vi "SP_Read_Sensor.vi"() -> ()   [LabVIEW 2013]
uses:
  <vilib>/event_ctls.llb/eventvkey.ctl
  Global_Not-Aus.vi
  <vilib>/Utility/file.llb/Write To Spreadsheet File (DBL).vi
  <vilib>/Utility/file.llb/Read From Spreadsheet File (string).vi
  Global_Start_Stop_Einzelschritt.vi
panel:
  in  "Stop Program":bool
  in  "Port for KOSY3":refnum<visa-resource-name>="COM2"
  in  "Port for Powersupply":refnum<visa-resource-name>="COM3"
  in  "Port for Write Head":refnum<visa-resource-name>="COM4"
  in  "Port for ED33":refnum<visa-resource-name>="COM7"
  in  "Port for ED32i":refnum<visa-resource-name>="COM8"
  in  "X,Y,Z Value Limits":T1={"mm Xmin "=0.0, "mm Xmax "=100.0, " mm Ymin "=0.0, "mm Ymax "=267.9, " mm Zmin"=0.0, "mm Zmax "=108.0, "Schritte oder mm Umin (0)"=0.0, "Schritte oder mm Umax (0)"=0.0, "Schritte oder mm Cmin (0)"=0.0, "Schritte oder mm Cmax (0)"=0.0, "Schritte oder mm Amin (0)"=0.0, "Schritte oder mm Amax (0)"=0.0, "Schritte oder mm Bmin (0)"=0.0, "Schritte oder mm Bmax (0)"=0.0}
  out "Error Out":errorcluster caption="error out"
  in  "Error In":errorcluster caption="error in"
  out "Movement":T2={"Axis"=36, "Direction(To/From)"=0, "Speed in mm/s\n (5)[0,025-20]"=5.0, "IV6"=FALSE} {"Direction(To/From)" items=["vom Endschalter weg", "zum Endschalter hin"]; "Speed in mm/s\n (5)[0,025-20]" min=0.025 max=20; "Axis" items=["X-Achse"=36, "Y-Achse"=37, "Z-Achse"=38, "U-Achse"=63]}
  out "Keyboard Press Display":cluster{"Speed(+/-)":i16, "Movement":T3}
  out "Steps":dbl
  out "Current Sequence":string[](array[string])
  in  "Clear Sequence":bool
  in  "Load Sequence":bool
  out "Sequence":string[][](array[string])
  in  "File  Select":path
  in  "Activate Sequence?":bool
  in  "Tab Control":enum32{"Page 2"}(tab)
  in  "Main Tab":enum32{"Page 1", "Page 2"}(tab)
  in  "Multiple Control":enum32{"Position", "Sensors", "Results"}(tab)
  out "P6":dbl[](array[numeric])
  out "P5":dbl[](array[numeric])
  out "P4":dbl[](array[numeric])
  out "P3":dbl[](array[numeric])
  out "P7":dbl[](array[numeric])
  out "P2":dbl[](array[numeric])
  out "P1":dbl[](array[numeric])
  out "P8":dbl[](array[numeric])
  out "P9":dbl[](array[numeric])
  out "P10":dbl[](array[numeric])
  in  "Go To":bool
  in  "Position":T4(ring)
  in  "Save":bool
  in  "Reset All":bool
  in  "Reset":bool
  in  "Import":bool
  in  "File Path":path=path "Y:/01_Projekte/EPN93031_Schreibplatz/8_Konstruktionsunterlagen/8.5_Software/COPY_KOSY Steuerung LabVIEW/1.New_Code_2014_2015/2Pole_strip_Position.txt"
  in  "Export":bool
  out "Speed":dbl(knob) scale=0.0..10.0
  in  "Z axis":enum16{"Up", "Down"}(ring)
  in  "Y axis":enum16{"Forward", "Backward"}(ring)
  in  "X axis":enum16{"Left", "Right"}(ring)
  in  "Move Steps":bool
  in  "Steps(mm)":dbl[](array[numeric]) min=0.0
  in  "Count":dbl
  in  "Move & Measure":bool
  in  "ED33 Active?":bool
  in  "ED32i Active?":bool
  in  "Clear Sensor Readings":bool
  out "ED33_output":string[][](array[string])
  out "ED32i_output":string[][](array[string])
  out "ED32i":cluster{"Array 4[0]":i32, "Array 4[1]":i32}(graph)
  out "ED33":i32[](graph)
  out "Operation Done":string="Initialise"
  out "Current Status":string="Initialise"
  out "Moving":bool
  out "Stopped":bool
  in  "Home Position":bool
  out "Current Cordinates":T5 {"Schritte B" format="%#.4g"; "Schritte A" format="%#.4g"; "Schritte C" format="%#.4g"; "Schritte U" format="%#.4g"; "Z axis" format="%#.4g"; "Y axis" format="%#.4g"; "X axis" format="%#.4g"}
  # "Com port info"
  # "Instructions\n                                              Manual Control\n1. Run the program.\n2. Select 'Initialise' to start the program from first \n     or 'Continue' to continue the ongoing process.\n3. Select 'Normal Operation'.\n\nPolestrip Positions\n1. If already positions are already saved, select the corresponding \n    file in 'File Path' and then click 'Import' to get the corresponding\n    positions displayed on the front panel. \n2. Set the 'Speed' using (+/-) for the movement.\n3. Select a position from the dropdown 'Position'and click 'Go To'.\n    Else, \n1. Set the 'Speed' using (+/-) for the movement.\n2. Set the length for movement in 'Steps(mm)'  in corresponding \n    axis and also the direction of travel in the selected axis. \n    Then press 'Move'.\n3. Once desired position is reached, select a position from the \n    dropdown 'Position' and click 'Save'.\n4. Once all positions are saved in front panel, select the file  to be \n     saved in 'File Path' and click 'Export' to save positions to a text file.\n5. Select a position from the dropdown 'Position' and \n    Click 'Reset' to clear individual position.\n6. Click 'Reset All' to clear all positions.\n \nSensor Readings\nContinuous measurement\n1.Activate the sensor to be read from 'Read Sensors' tab.\n2.Set the length for movement in 'Steps(mm)' in corresponding \n    axis and also the direction of travel in the selected axis. \n    Then press 'Move'.\nMove and Measure\n1. Activate the sensor to be read from 'Read Sensors' tab.\n2.Set 'Count' to the number of times to measure.\n2.Set the length for movement in 'Steps(mm)' in corresponding \n    axis and also the direction of travel in the selected axis. \n    Then press 'Move Measure'.\n\n1. Click 'Clear' in 'Read Sensors' tab to clear the sensor readings.\n\n                                          Automatic Execution\n1. Run the program.\n2. Select 'Initialise' to start the program from first \n     or 'Continue' to continue the ongoing process.\n3. Select 'Normal Operation'.\n4. Select the corresponding file in 'File Select' and then click 'Load' \n    to get the corresponding codes in 'Sequence' .\n5. Click 'Clear' to clear sequence.\n6. Click 'Activate Sequence?' to run the automatic execution. \n\n                                                       General\n1. Click 'Stop Program' to stop the running program.\n2. Click 'Home Position' to take the write head to (0,0,0)."
  # "Instructions\n\n1. Positions are already saved, select the file in 'File Path' \n    and then 'Import' to get the positions displayed . \n2. Set the 'Speed' using (+/-) for the movement.\n3. Select a 'Position'and click 'Go To'.\n4. Click 'Reset All' to reset all positions and \n     'Import' again."
  # "Polestrip Positions"
  # "Instructions\n\nContinuous measurement\n1.Activate the sensor to be read.\n2.Set the length for movement in 'Steps(mm)' in corresponding \n    axis and also the direction of travel in the selected axis. \n    Then press 'Move'.\nMove and Measure\n1. Activate the sensor to be read.\n2.Set the length for movement in 'Steps(mm)' in corresponding \n    axis and also the direction of travel in the selected axis. \n3. Set 'Count' to the number of times to measure.  \n    Then press 'Move Measure'."
  # "[Click 'Clear' in 'Read Sensors' tab to clear the sensor readings.]"
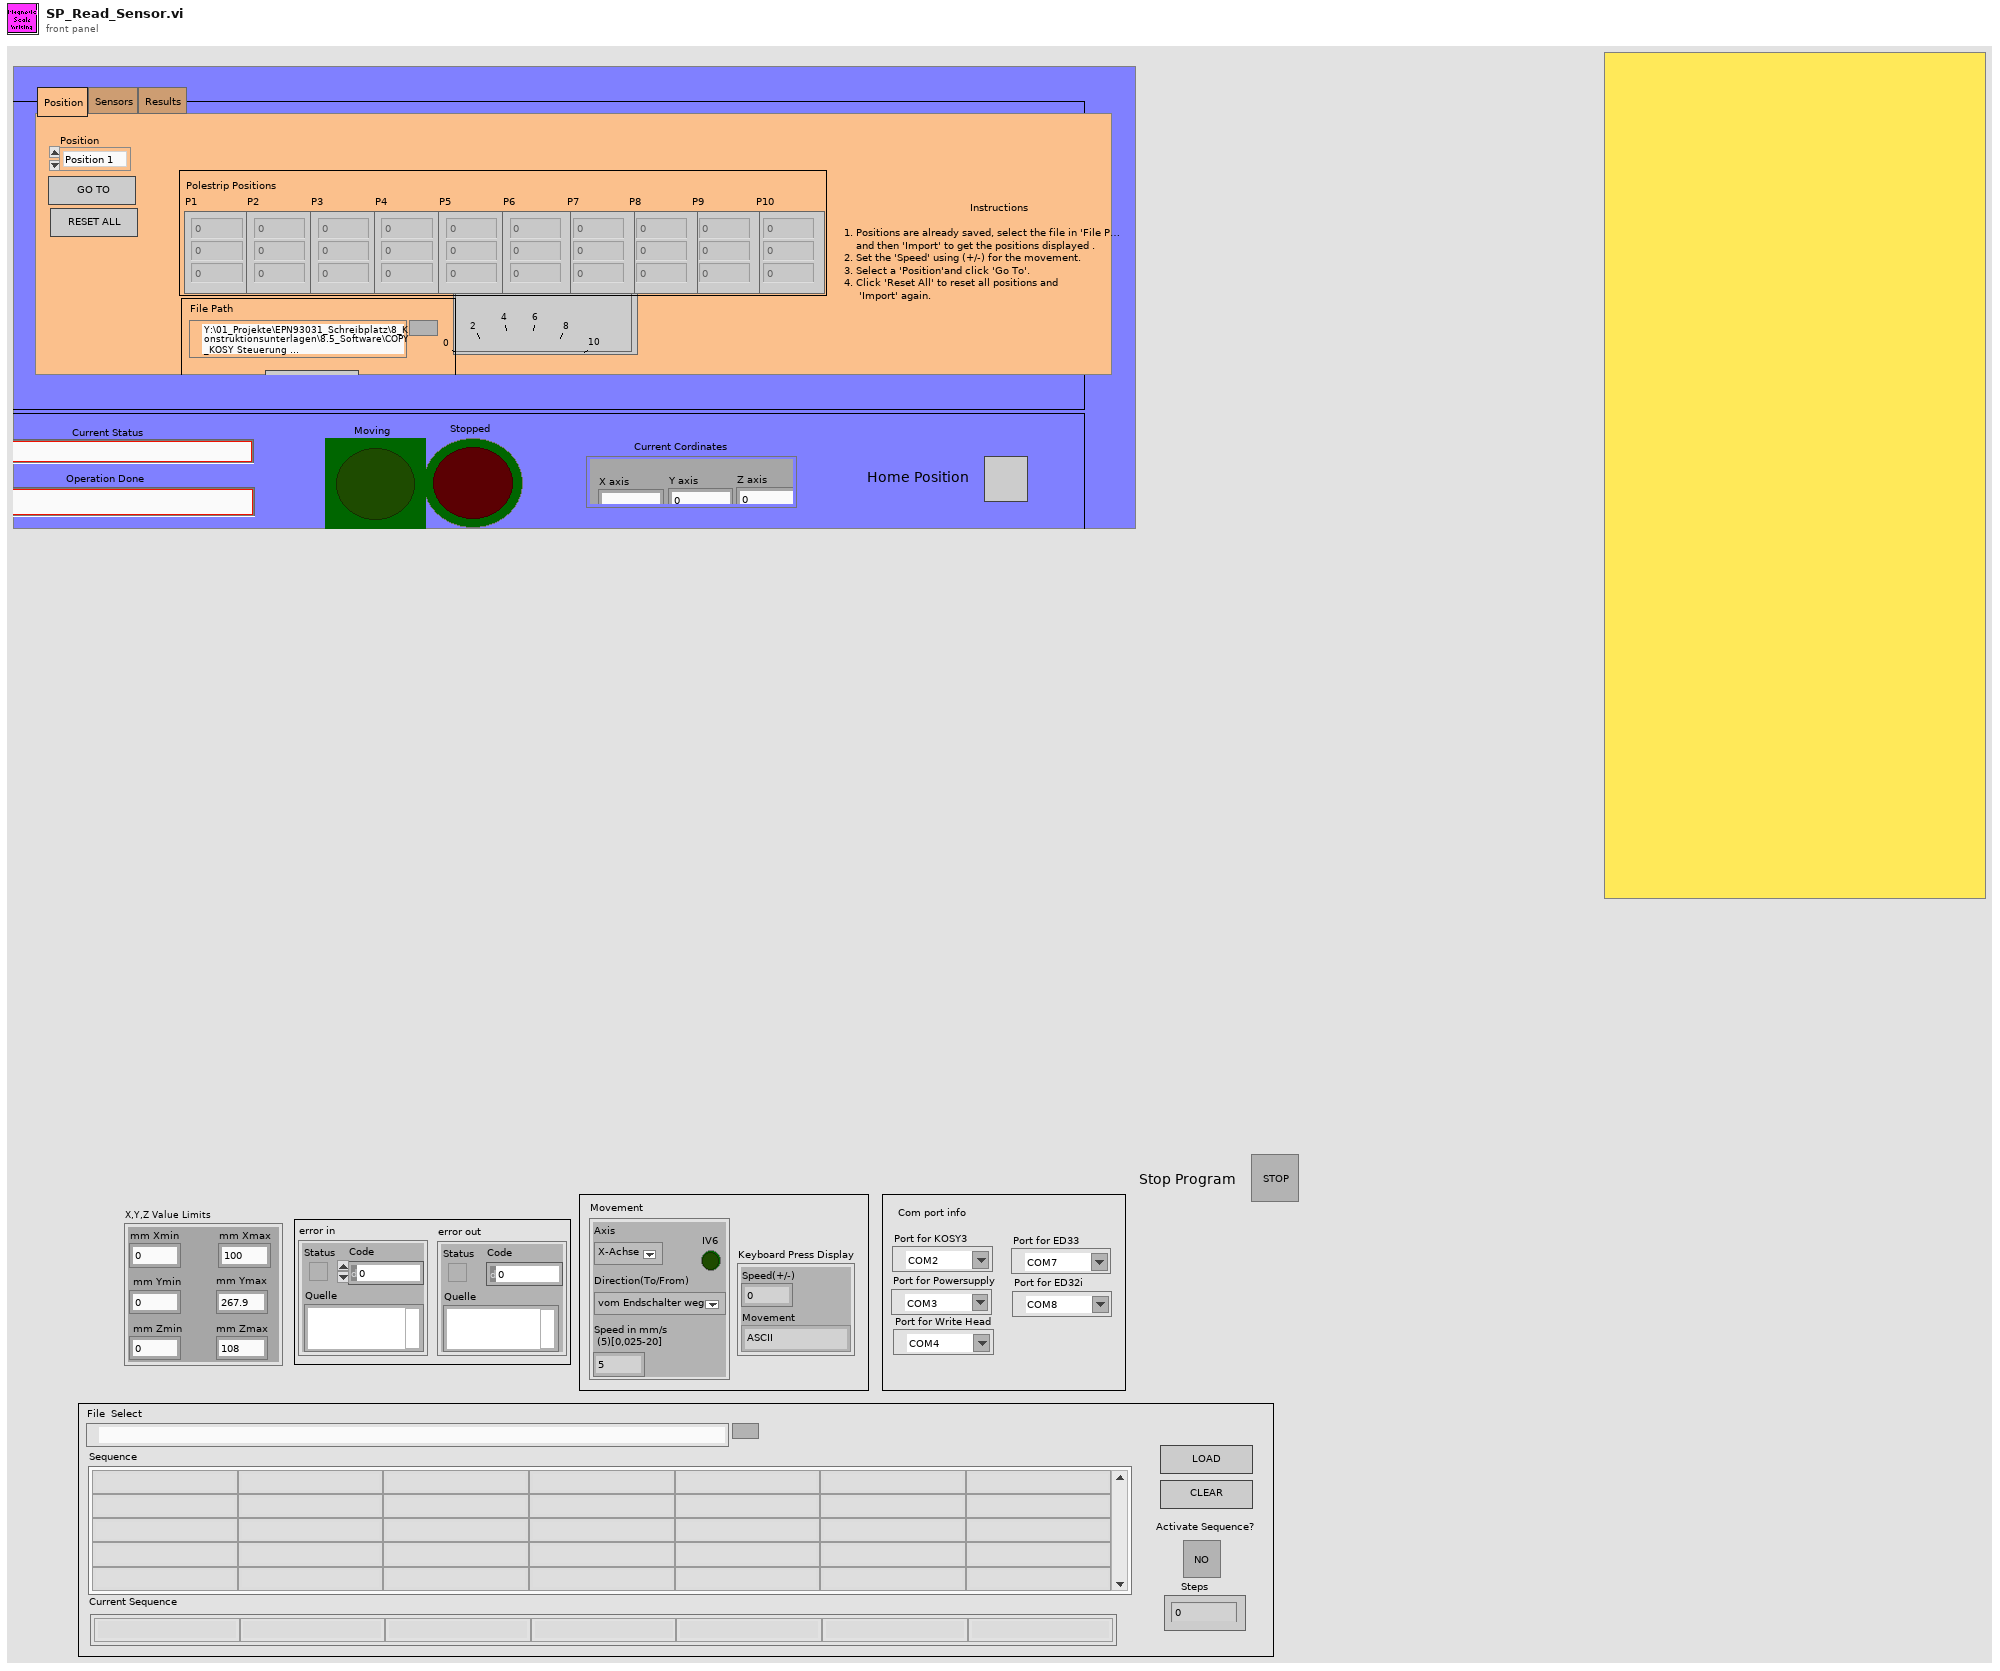
[diagram p1: front panel]
types:
  T1 = cluster{"mm Xmin ":sgl, "mm Xmax ":sgl, " mm Ymin ":sgl, "mm Ymax ":sgl, " mm Zmin":sgl, "mm Zmax ":sgl, "Schritte oder mm Umin (0)":sgl, "Schritte oder mm Umax (0)":sgl, "Schritte oder mm Cmin (0)":sgl, "Schritte oder mm Cmax (0)":sgl, "Schritte oder mm Amin (0)":sgl, "Schritte oder mm Amax (0)":sgl, "Schritte oder mm Bmin (0)":sgl, "Schritte oder mm Bmax (0)":sgl}
  T2 = cluster{"Axis":u8, "Direction(To/From)":u8, "Speed in mm/s\n (5)[0,025-20]":sgl, "IV6":bool}
  T3 = typedef "eventvkey.ctl" = enum16{"ASCII", "Enter", "Return", "Shift", "Ctrl", "Alt", "Cmd", "Opt", "Caps", "NumLock", "Clear", "Break", "Up", "Down", "Left", "Right", "Insert", "Delete", "Home", "End", "PageUp", "PageDown", "Escape", "Help", "Pause", "ScrollLock", "F1", "F2", "F3", "F4", "F5", "F6", "F7", "F8", "F9", "F10", "F11", "F12", "F13", "F14", "F15", "F16", "F17", "F18", "F19", "F20", "F21", "F22", "F23", "F24", "Play", "VolumeUp", "VolumeDown", "Mute", "Two Byte Char"}
  T4 = enum16{"Position 1", "Position 2", "Position 3", "Position 4", "Position 5", "Position 6", "Position 7", "Position 8", "Position 9", "Position 10"}
  T5 = cluster{"X axis":sgl, "Y axis":sgl, "Z axis":sgl, "Schritte U":sgl, "Schritte C":sgl, "Schritte A":sgl, "Schritte B":sgl}
  T6 = enum32{"Page Enabled", "Page Disabled", "Page Disabled & Grayed"}
  T7 = cluster{"Geschwindigkeit X in mm/s\n(5) [0,025-15]":sgl, "Geschwindigkeit Y in mm/s\n(5) [0,025-15]":sgl, "Geschwindigkeit Z in mm/s\n(5) [0,025-15]":sgl, "GeschwindigkeitU in mm/s\n(5) [0,025-15]":sgl}
  T8 = cluster{"Schritte X":sgl, "Schritte Y":sgl, "Schritte Z":sgl, "Schritte U":sgl, "Schritte C":sgl, "Schritte A":sgl, "Schritte B":sgl}
  T9 = cluster{"[0]":dbl, "[1]":dbl, "[2]":dbl, "[3]":dbl, "[4]":dbl, "[5]":dbl, "[6]":dbl, "[7]":dbl, "[8]":dbl}
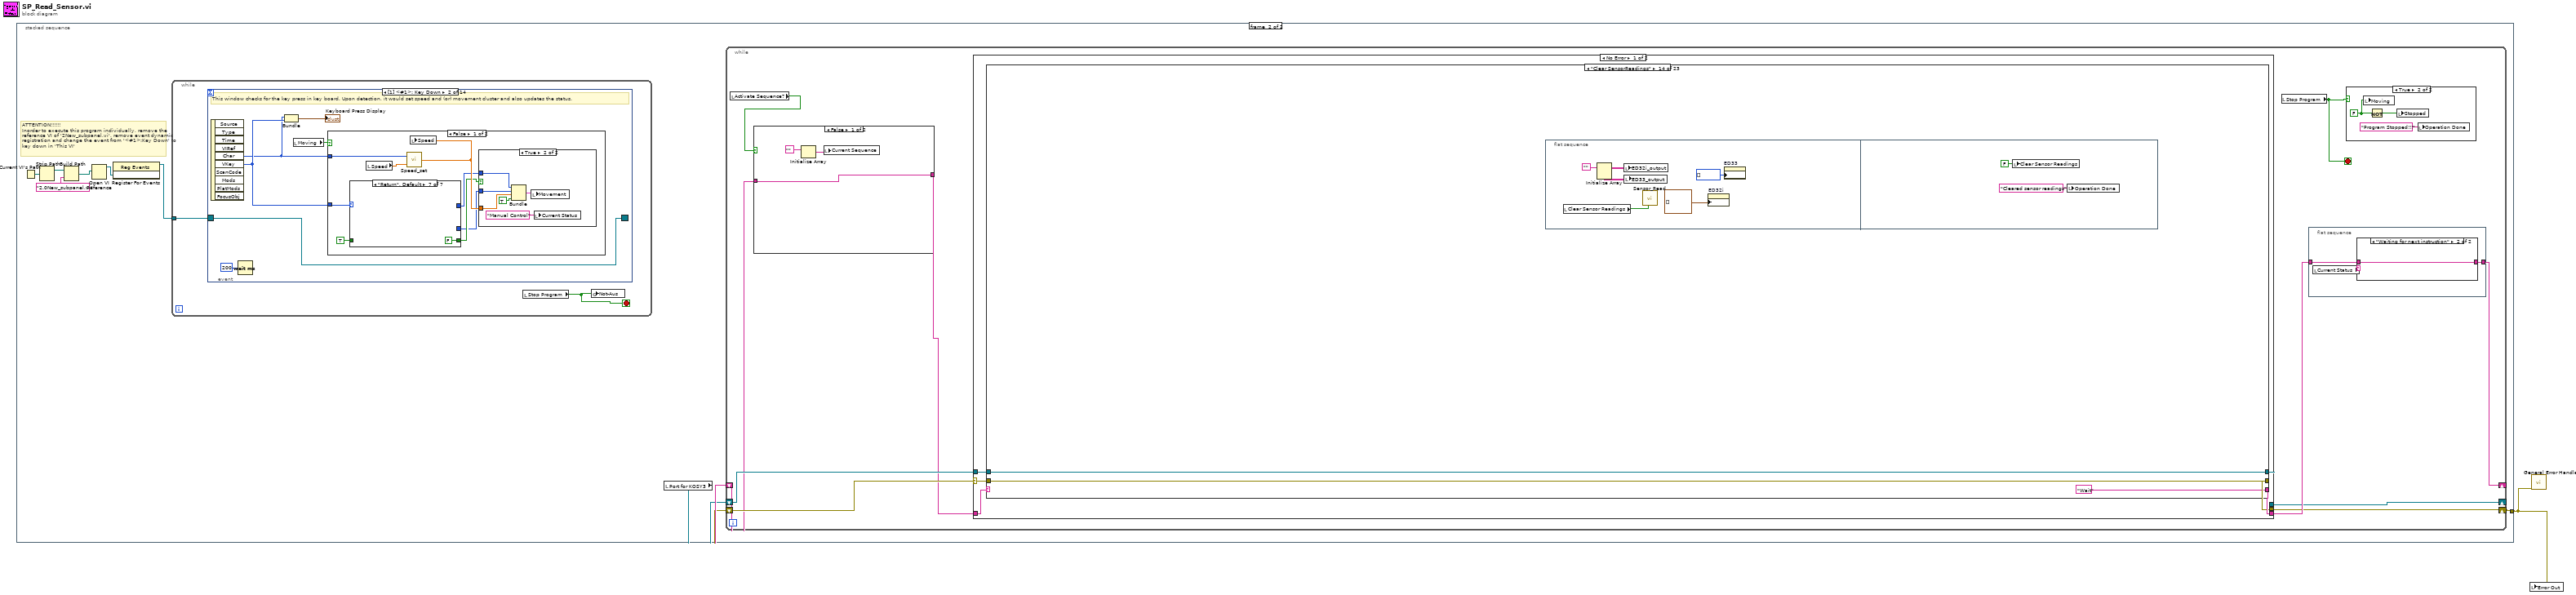
[diagram p0: block diagram]
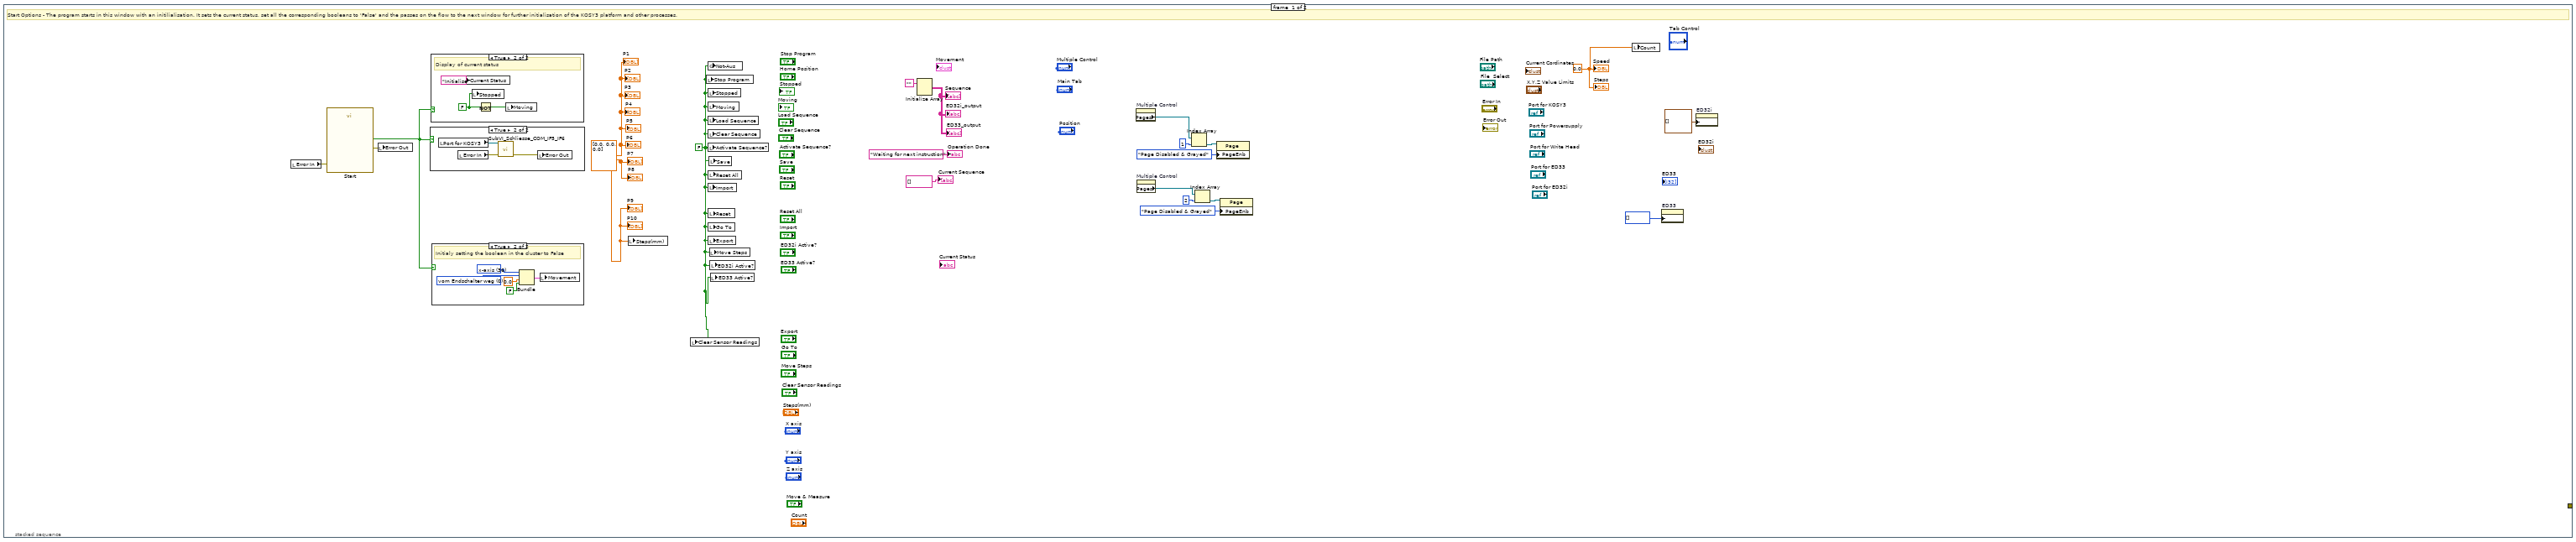
[diagram p2: hidden frame]
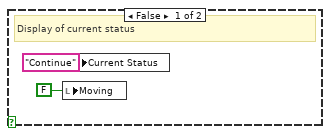
[diagram p5: hidden frame]
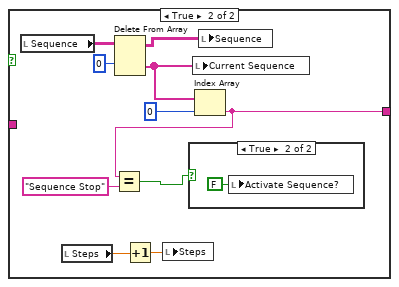
[diagram p6: hidden frame]
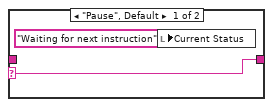
[diagram p9: hidden frame]
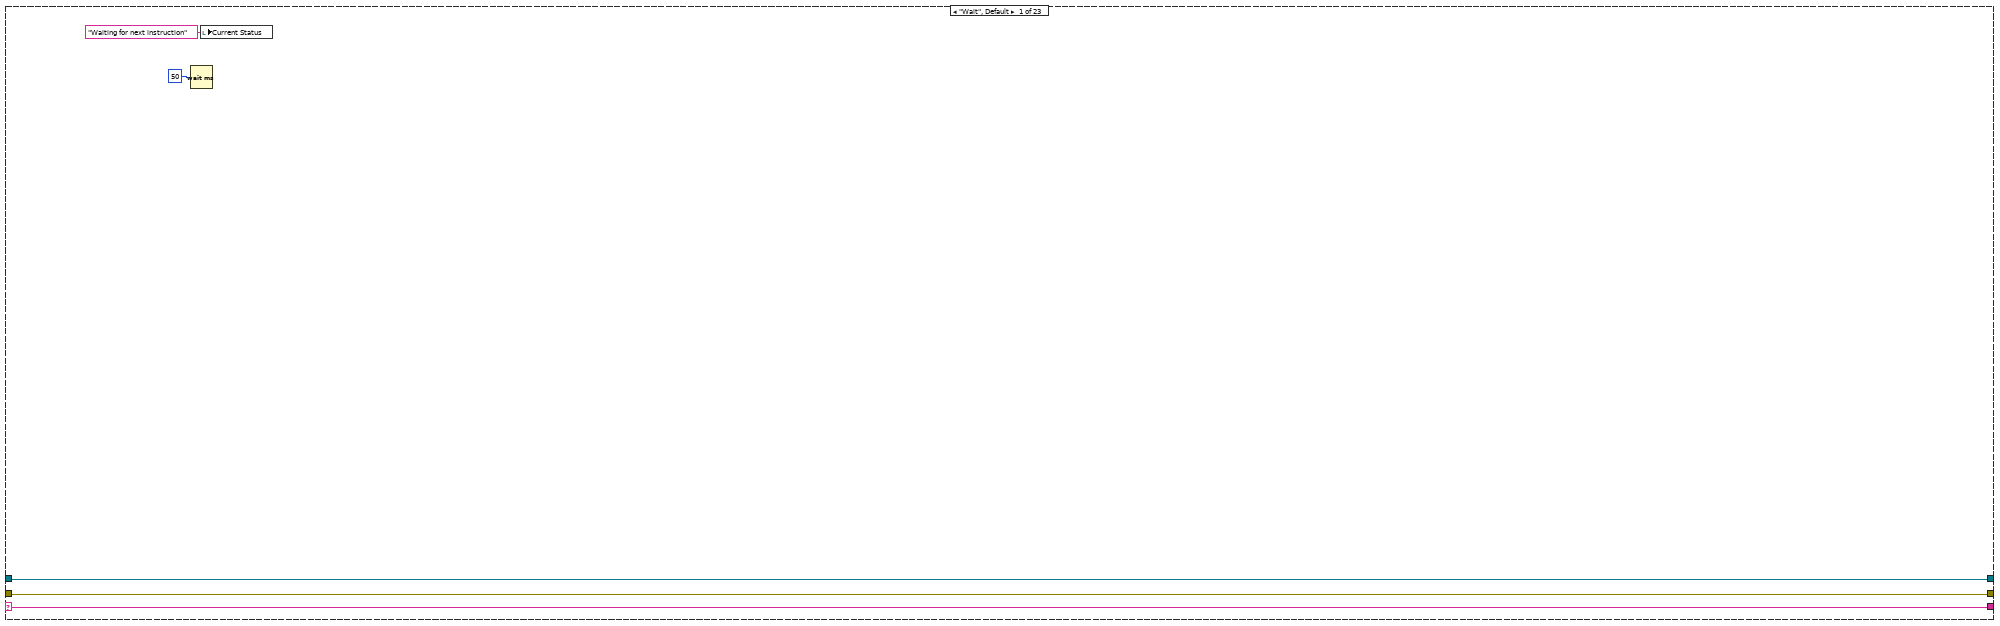
[diagram p10: hidden frame]
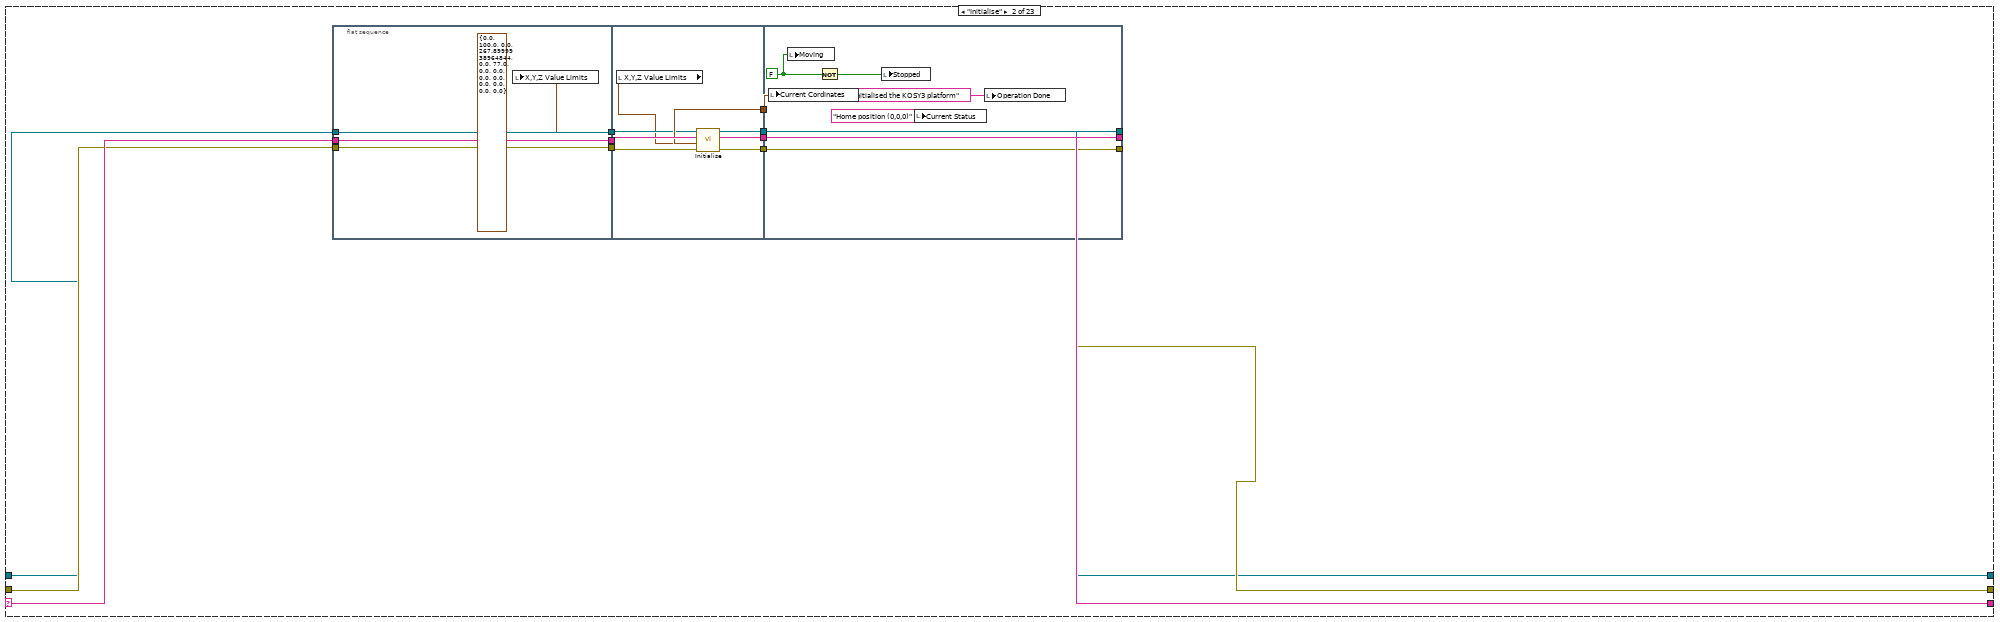
[diagram p11: hidden frame]
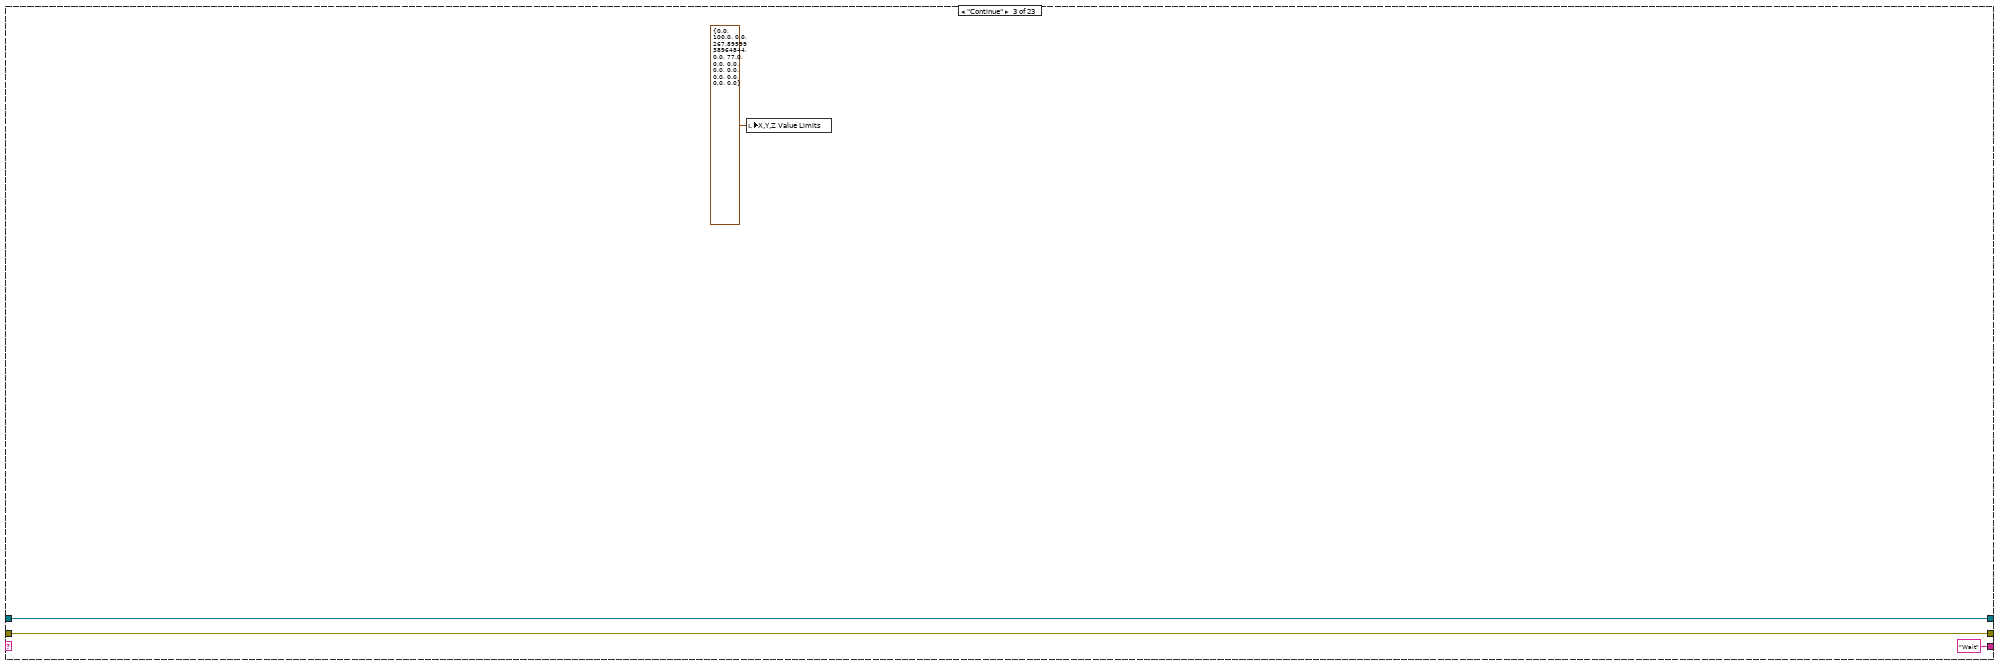
[diagram p12: hidden frame]
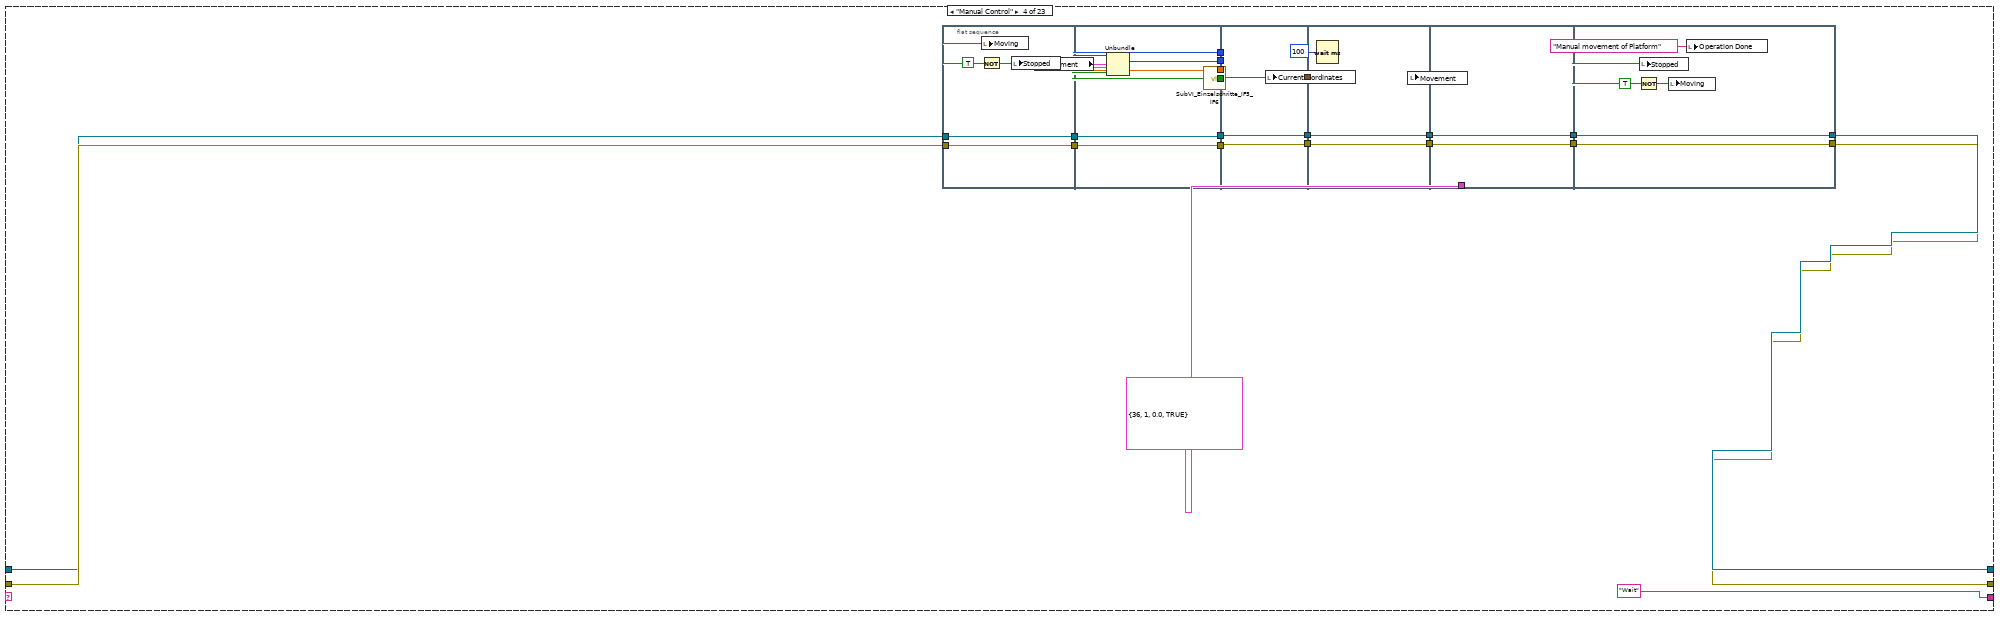
[diagram p13: hidden frame]
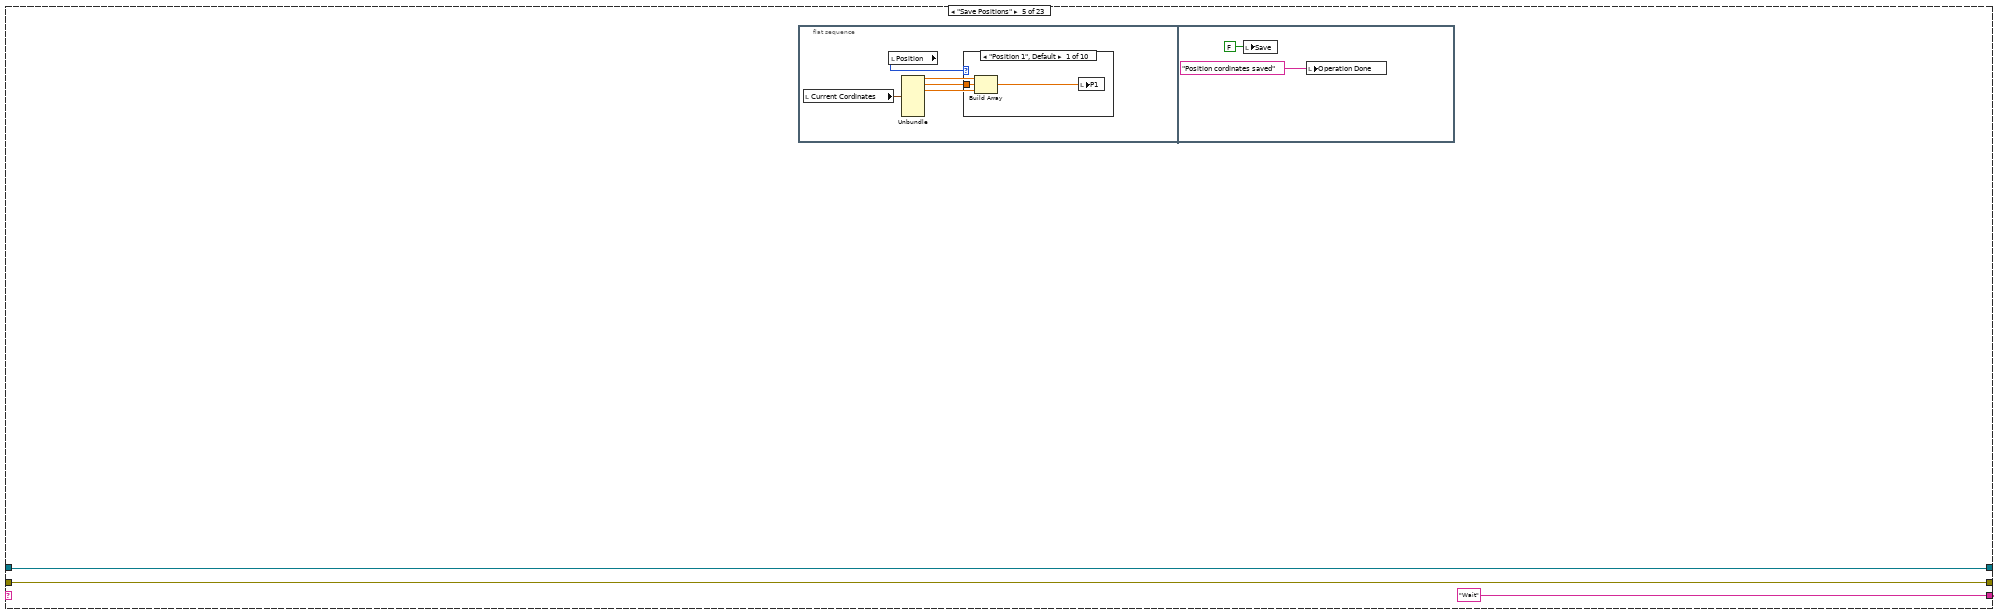
[diagram p14: hidden frame]
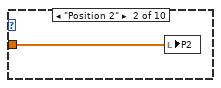
[diagram p15: hidden frame]
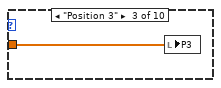
[diagram p16: hidden frame]
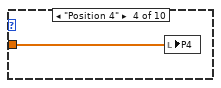
[diagram p17: hidden frame]
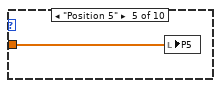
[diagram p18: hidden frame]
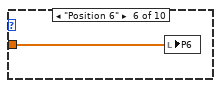
[diagram p19: hidden frame]
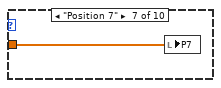
[diagram p20: hidden frame]
diagram:
  n1 = stacked-sequence {
    tunnel: [_ w41] -> w1
    frame #0 {
      w10 = 0.0 ("Speed")
      w11 = dbl[] [0.0, 0.0, 0.0] ("P1")
      w14 = FALSE ("Moving")
      # "Start Options - The program starts in this window with an initilialisation. It sets the current status, set all the corresponding booleans to 'False' and the passes on the flow to the next window for further initialisation of the KOSY3 platform and other processes."
      n2 = local read "Error In"() -> (w21:errorcluster)
      n3 = call "Start"("error in (no error)"=w21) -> ("Initialise"=w19:bool, "error out"=w20:errorcluster)  [unwired: 17 in]
      n4 = local write "Error Out"(w20) -> ()
      n5 = case shown="True" w19 {
        frame False {
        }
        frame True {
          n6 = local read "Port for KOSY3"() -> (w24:refnum<visa-resource-name>)
          n7 = local read "Error In"() -> (w23:errorcluster)
          n8 = call "SubVI_Schliesse_COM_IF5_IF6.vi"("VISA resource name in"=w24, "error in"=w23) -> ("error out"=w22:errorcluster)  [unwired: 13 in]
          n9 = local write "Error Out"(w22) -> ()
        }
      }
      n10 = case shown="True" w19 {
        frame False {
          # "Display of current status"
          n11 = local write "Moving"(FALSE ("Stopped")) -> ()
          n12 = local write "Current Status"("Continue") -> ()
        }
        frame True {
          w32 = FALSE ("Stopped")
          # "Display of current status"
          n13 = local write "Current Status"("Initialise") -> ()
          n14 = local write "Stopped"(w32) -> ()
          n15 = Not(x=w32) -> (.not. x?=w33:bool)
          n16 = local write "Moving"(w33) -> ()
        }
      }
      n17 = case shown="True" w19 {
        frame False {
        }
        frame True {
          w28 = u16 0 items=["vom Endschalter weg", "zum Endschalter hin"]
          w29 = u16 36 items=["x-axis"=36, "y-axis"=37, "z-axis"=38]
          # "Initialy setting the boolean in the cluster to False"
          n18 = Bundle(w29, w28, 0.0, FALSE) -> (w25:cluster{u16, u16, dbl, bool})  [unwired: 1 in]
          n19 = local write "Movement"(w25) -> ()
        }
      }
      n20 = local write "Steps(mm)"(w11) -> ()
      n21 = local write "Clear Sensor Readings"(w14) -> ()
      n22 = local write "Stop Program"(w14) -> ()
      n23 = global write "Global_Not-Aus.vi" "Not-Aus"(w14) -> ()
      n24 = local write "Stopped"(w14) -> ()
      n25 = local write "Moving"(w14) -> ()
      n26 = local write "Load Sequence"(w14) -> ()
      n27 = local write "Clear Sequence"(w14) -> ()
      n28 = local write "Activate Sequence?"(w14) -> ()
      n29 = local write "Import"(w14) -> ()
      n30 = local write "Reset All"(w14) -> ()
      n31 = local write "Reset"(w14) -> ()
      n32 = local write "Go To"(w14) -> ()
      n33 = local write "Export"(w14) -> ()
      n34 = local write "Save"(w14) -> ()
      n35 = local write "Move Steps"(w14) -> ()
      n36 = local write "ED32i Active?"(w14) -> ()
      n37 = local write "ED33 Active?"(w14) -> ()
      n38 = Initialize Array("" ("element")) -> (→"Sequence" →"ED32i_output" →"ED33_output":string[][])  [unwired: 2 in]
      n39 = property on="Multiple Control" class="TabCtl (strict)"() -> ("Pages"=w6:refnum<vi>[])  [unwired: 2 in, 2 out]
      n40 = property on="Multiple Control" class="TabCtl (strict)"() -> ("Pages"=w2:refnum<vi>[])  [unwired: 2 in, 2 out]
      n41 = Index Array(array=w6, index=1) -> (element=w7:refnum<vi>)
      n42 = Index Array(array=w2, index=2) -> (element=w3:refnum<vi>)
      n43 = property class="Page"(reference=w7, "PageEnb"=T6."Page Disabled & Grayed" ("Page Enabled State")) -> ()  [unwired: 1 in, 2 out]
      n44 = property class="Page"(reference=w3, "PageEnb"=T6."Page Disabled & Grayed" ("Page Enabled State")) -> ()  [unwired: 1 in, 2 out]
      n45 = local write "Count"(w10) -> ()
      n46 = property on="ED33" class="WFChart (strict)"("History Data"=i32[] []) -> ()  [unwired: 2 in, 2 out]
      n47 = property on="ED32i" class="WFChart (strict)"("History Data"=cluster{"Array 4[0]":i32, "Array 4[1]":i32}[] []) -> ()  [unwired: 2 in, 2 out]
      "Speed" <- w10
      "P1" <- w11
      "P2" <- w11
      "P3" <- w11
      "P7" <- w11
      "P4" <- w11
      "P5" <- w11
      "P6" <- w11
      "P8" <- w11
      "P9" <- w11
      "P10" <- w11
      "Current Sequence" <- string[] [] ("Current Sequence")
      "Operation Done" <- "Waiting for next instruction" ("Operation Done")
      "Steps" <- w10
    }
    frame #1 {
      # "ATTENTION!!!!!!\nInorder to execute this program individually, remove the reference VI of '2New_subpanel.vi', remove event dynamic registration and change the event from '<#1>:Key Down' to key down in 'This VI'"
      n48 = Current VI's Path() -> (path=w39:path)
      n49 = Strip Path(path=w39) -> (stripped path=w38:path)  [unwired: 1 out]
      n50 = Build Path(base path=w38, name or relative path="2.0New_subpanel.vi") -> (appended path=w36:path)
      n51 = Open VI Reference(vi path=w36) -> (vi reference=w40:refnum<vi>)  [unwired: 5 in, 1 out]
      n52 = register-events(w40) -> (reference out=w35:refnum<event-registration>)  [unwired: 2 in, 1 out]
      n53 = while {
        tunnel: w35 -> [w716]
        stop <- w717 stop-if-true
        n54 = event shown="[1] <#1>: Key Down" {
          selector: w716 -> [_ w719 _ _ _ _ _ _ _ _ _ _ _ _]
          dyn-events: [_ w719 _ _ _ _ _ _ _ _ _ _ _ _] -> _
          timeout: _ -> [_ _ _ _ _ _ _ _ _ _ _ _ _ _]
          event Timeout {
            n55 = event-data() -> ()  [unwired: 1 in, 2 out]
            n56 = global write "Global_Start_Stop_Einzelschritt.vi" "Boolesch"(FALSE ("Boolesch")) -> ()
          }
          event Key Down {
            # "This window checks for the key press in key board. Upon detection, it would set speed and (or) movement cluster and also updates the status."
            n57 = event-data() -> ("Char"=w720:i16, "VKey"=w722:T3)  [unwired: 1 in, 8 out]
            n58 = Wait (ms)(milliseconds to wait=u32 200) -> ()  [unwired: 1 out]
            n59 = Bundle("Char"=w720, "VKey"=w722) -> (→"Keyboard Press Display":cluster{"Char":i16, "VKey":T3})  [unwired: 1 in]
            n60 = local read "Moving"() -> (w724:bool)
            n61 = case shown="False" w724 {
              tunnel: w722 -> [w730 _]
              tunnel: w720 -> [w732 _]
              frame False {
                n62 = case shown="\"Return\", Default" w730 {
                  tunnel: [w733 w736 w739 w742 w745 w748 FALSE] -> w729
                  tunnel: [w735 w738 w741 w744 w747 w750 _] -> w727
                  tunnel: [w734 w737 w740 w743 w746 w749 _] -> w726
                  tunnel: TRUE -> [w733 w736 w739 w742 w745 w748 _]
                  frame "Left" {
                    w734 = u16 1 items=["vom Endschalter weg", "zum Endschalter hin"]
                    w735 = u16 36 items=["x-axis"=36, "y-axis"=37, "z-axis"=38]
                    # "Direction control(VKey identifies the directional keys)"
                  }
                  frame "Right" {
                    w737 = u16 0 items=["vom Endschalter weg", "zum Endschalter hin"]
                    w738 = u16 36 items=["x-axis"=36, "y-axis"=37, "z-axis"=38]
                    # "Direction control"
                  }
                  frame "Up" {
                    w740 = u16 1 items=["vom Endschalter weg", "zum Endschalter hin"]
                    w741 = u16 37 items=["x-axis"=36, "y-axis"=37, "z-axis"=38]
                    # "Direction control"
                  }
                  frame "Down" {
                    w743 = u16 0 items=["vom Endschalter weg", "zum Endschalter hin"]
                    w744 = u16 37 items=["x-axis"=36, "y-axis"=37, "z-axis"=38]
                  }
                  frame "PageUp" {
                    w746 = u16 1 items=["vom Endschalter weg", "zum Endschalter hin"]
                    w747 = u16 38 items=["x-axis"=36, "y-axis"=37, "z-axis"=38]
                  }
                  frame "PageDown" {
                    w749 = u16 0 items=["vom Endschalter weg", "zum Endschalter hin"]
                    w750 = u16 38 items=["x-axis"=36, "y-axis"=37, "z-axis"=38]
                  }
                  frame "Return", Default {
                  }
                }
                n63 = local read "Speed"() -> (w725:dbl)
                n64 = call "Speed_set.vi"("Speed"=w725, "Char"=w732) -> ("Speed"=w731:dbl)
                n65 = local write "Speed"(w731) -> ()
                n66 = case shown="True" w729 {
                  tunnel: w731 -> [_ w755]
                  tunnel: w727 -> [_ w754]
                  tunnel: w726 -> [_ w753]
                  frame False {
                  }
                  frame True {
                    n67 = Bundle(w754, w753, "Speed"=w755, TRUE) -> (w752:cluster{u16, u16, "Speed":dbl, bool})  [unwired: 1 in]
                    n68 = local write "Movement"(w752) -> ()
                    n69 = local write "Current Status"("Manual Control" ("Status")) -> ()
                  }
                }
              }
              frame True {
                n70 = global write "Global_Start_Stop_Einzelschritt.vi" "Boolesch"(TRUE) -> ()
                n71 = local write "Moving"(FALSE) -> ()
              }
            }
          }
          event "Home Position": Value Change {
            # "This window corresponds to the 'Home position' button on the Front Panel. Pressing the button will take KOSY3 paltform to the home position (0,0,0)"
            n72 = event-data() -> ()  [unwired: 1 in, 6 out]
            n73 = local write "Current Status"("Home Position" ("Status")) -> ()
          }
          event "Save": Value Change {
            # "When the 'SAVE' button in the Front Panel is pressed, it would save the current cordinates of the KOSY3 platform to the selected position."
            n74 = event-data() -> ()  [unwired: 1 in, 6 out]
            n75 = local write "Current Status"("Save Positions" ("Status")) -> ()
          }
          event "Reset": Value Change {
            # "When 'RESET' in the Front Panel is pressed, it resets the cordinates in the selected position to (0,0,0)"
            n76 = event-data() -> ()  [unwired: 1 in, 6 out]
            n77 = local write "Current Status"("Reset Position" ("Status")) -> ()
          }
          event "Reset All": Value Change {
            # "When 'RESET ALL' in the Front Panel is pressed, it resets the cordinates in all positions to (0,0,0)"
            n78 = event-data() -> ()  [unwired: 1 in, 6 out]
            n79 = local write "Current Status"("Reset All" ("Status")) -> ()
          }
          event "Go To": Value Change {
            n80 = event-data() -> ()  [unwired: 1 in, 6 out]
            n81 = local write "Current Status"("Go Position" ("Status")) -> ()
          }
          event "Move Steps": Value Change {
            n82 = event-data() -> ()  [unwired: 1 in, 6 out]
            n83 = local write "Current Status"("Go Straight" ("Status")) -> ()
          }
          event "Move & Measure": Value Change {
            n84 = event-data() -> ()  [unwired: 1 in, 6 out]
            n85 = local write "Current Status"("Move & Measure" ("Status")) -> ()
          }
          event "Import": Value Change {
            n86 = event-data() -> ()  [unwired: 1 in, 6 out]
            n87 = local write "Current Status"("Import Cordinates" ("Status")) -> ()
          }
          event "Export": Value Change {
            n88 = event-data() -> ()  [unwired: 1 in, 6 out]
            n89 = local write "Current Status"("Export Cordinates" ("Status")) -> ()
          }
          event "Load Sequence": Value Change {
            n90 = event-data() -> ()  [unwired: 1 in, 6 out]
            n91 = local write "Current Status"("Load Sequence" ("Status")) -> ()
          }
          event "Clear Sequence": Value Change {
            n92 = event-data() -> ()  [unwired: 1 in, 6 out]
            n93 = local write "Current Status"("Clear Sequence" ("Status")) -> ()
          }
          event "Clear Sensor Readings": Value Change {
            n94 = event-data() -> ()  [unwired: 1 in, 6 out]
            n95 = local write "Current Status"("Clear SensorReadings" ("Status")) -> ()
          }
        }
        n96 = local read "Stop Program"() -> (w717:bool)
        n97 = global write "Global_Not-Aus.vi" "Not-Aus"(w717) -> ()
      }
      n98 = local read "Port for KOSY3"() -> (w42:refnum<visa-resource-name>)
      n99 = local read "Current Status"() -> (w44:string)
      n100 = local read "Error In"() -> (w43:errorcluster)
      n101 = while {
        shift-right: [w48] -> w41
        shift-left: w43 -> [w54]
        shift-right: [w49] -> _
        shift-left: w42 -> [w50]
        shift-right: [w52] -> _
        shift-left: w44 -> [w47]
        stop <- w51 stop-if-true
        n102 = local read "Activate Sequence?"() -> (w45:bool)
        n103 = case shown="False" w45 {
          tunnel: w47 -> [w57 _]
          tunnel: [w57 w62] -> w46
          frame False {
            n104 = Initialize Array("") -> (w55:string[])  [unwired: 1 in]
            n105 = local write "Current Sequence"(w55) -> ()
          }
          frame True {
            n106 = local read "Sequence"() -> (w67:string[][])
            n107 = local read "Steps"() -> (w59:dbl)
            n108 = Delete From Array(array=w67, index (row)=0) -> (deleted portion=w64:string[], array with subset deleted=w65:string[][])  [unwired: 2 in]
            n109 = Increment(x=w59) -> (x+1=w58:dbl)
            n110 = local write "Steps"(w58) -> ()
            n111 = local write "Current Sequence"(w64) -> ()
            n112 = Index Array(array=w64, index=0) -> (element=w62:string)
            n113 = Equal?(x=w62, y="Sequence Stop") -> (x = y?=w60:bool)
            n114 = case shown="True" w60 {
              frame False {
              }
              frame True {
                n115 = local write "Activate Sequence?"(FALSE ("Activate Sequence?")) -> ()
              }
            }
            n116 = local write "Sequence"(w65) -> ()
          }
        }
        n117 = case shown="No Error" w54 {
          selector: w54 -> [w80 w711]
          tunnel: w46 -> [w83 _]
          tunnel: [w82 "Error" ("String 2")] -> w53
          tunnel: w50 -> [w81 w712]
          tunnel: [w78 w712] -> w49
          tunnel: [w79 w711] -> w48
          frame No Error {
            n118 = case shown="\"Clear SensorReadings\"" w83 {
              selector: w83 -> [w87 w101 _ _ _ _ _ _ _ _ _ _ _ _ _ _ _ _ _ _ _ _ _]
              tunnel: [w87 w98 "Wait" ("String 2") "Wait" "Wait" ("String 2") "Wait" ("String 2") "Wait" ("String 2") "Wait" ("String 2") "Wait" ("String 2") "Wait" ("String 2") "Wait" ("String 2") "Wait" ("String 2") "Wait" ("String 2") "Wait" ("String 2") "Wait" ("String 2") "Wait" ("String 2") "Wait" ("String 2") "Wait" ("String 2") "Wait" ("String 2") "Wait" ("String 2") "Wait" ("String 2") "Wait" ("String 2") "Wait" ("String 2")] -> w82
              tunnel: w81 -> [w84 w96 w124 w134 w180 w201 w218 w230 w268 w284 w323 w346 w353 w362 w371 w380 w394 w429 w556 w585 w593 w696 w703]
              tunnel: w80 -> [w85 w97 w122 w137 w179 w200 w217 w229 w269 w285 w325 w347 w354 w361 w372 w379 w395 w430 w554 w584 w594 w695 w705]
              tunnel: [w85 w94 w122 w129 w179 w200 w217 w227 w269 w285 w320 w347 w354 w361 w372 w379 w396 w428 w554 w584 w594 w695 w704] -> w79
              tunnel: [w84 w92 w124 w133 w180 w201 w218 w228 w268 w284 w322 w346 w353 w362 w371 w380 w397 w427 w556 w585 w592 w696 w703] -> w78
              frame "Wait", Default {
                n119 = Wait (ms)(milliseconds to wait=50) -> ()  [unwired: 1 out]
                n120 = local write "Current Status"("Waiting for next instruction" ("Status")) -> ()
              }
              frame "Initialise" {
                n121 = flat-sequence {
                  tunnel: w96 -> [w103]
                  tunnel: w97 -> [w104]
                  tunnel: w101 -> [w105]
                  tunnel: [w105] -> w91
                  tunnel: [w104] -> w90
                  tunnel: [w103] -> w89
                  tunnel: [w112] -> w100
                  tunnel: [w111] -> w99
                  tunnel: [w108] -> w95
                  tunnel: [w107] -> w93
                  tunnel: w91 -> [w113]
                  tunnel: w90 -> [w110]
                  tunnel: w89 -> [w109]
                  tunnel: w100 -> [w118]
                  tunnel: w99 -> [w117]
                  tunnel: [w117] -> w98
                  tunnel: [w115] -> w92
                  tunnel: w95 -> [w115]
                  tunnel: [w114] -> w94
                  tunnel: w93 -> [w114]
                  frame #0 {
                    n122 = local write "X,Y,Z Value Limits"(T1 {"mm Xmin "=0.0, "mm Xmax "=100.0, " mm Ymin "=0.0, "mm Ymax "=267.9, " mm Zmin"=0.0, "mm Zmax "=77.0, "Schritte oder mm Umin (0)"=0.0, "Schritte oder mm Umax (0)"=0.0, "Schritte oder mm Cmin (0)"=0.0, "Schritte oder mm Cmax (0)"=0.0, "Schritte oder mm Amin (0)"=0.0, "Schritte oder mm Amax (0)"=0.0, "Schritte oder mm Bmin (0)"=0.0, "Schritte oder mm Bmax (0)"=0.0} ("X,Y,Z Value Limits")) -> ()
                  }
                  frame #1 {
                    n123 = local read "X,Y,Z Value Limits"() -> (w106:T1)
                    n124 = call "Initialise.vi"("error IO"=w110, "X,Y,Z values"=w106, "String"=w113, "Port for KOSY3"=w109) -> ("Fehler (Ausgang)"=w107:errorcluster, "Cordinates of the  KOSY3 Platform"=w112:T8, "String 2"=w111:string, "VISA-Referenz (Ausgang)"=w108:refnum<visa-resource-name>)
                  }
                  frame #2 {
                    w119 = FALSE ("Stopped")
                    n125 = local write "Current Cordinates"(w118) -> ()
                    n126 = local write "Moving"(w119) -> ()
                    n127 = Not(x=w119) -> (.not. x?=w120:bool)
                    n128 = local write "Stopped"(w120) -> ()
                    n129 = local write "Current Status"("Home position (0,0,0)" ("Status")) -> ()
                    n130 = local write "Operation Done"("Initialised the KOSY3 platform" ("Operation Done")) -> ()
                  }
                }
              }
              frame "Continue" {
                n131 = local write "X,Y,Z Value Limits"(T1 {"mm Xmin "=0.0, "mm Xmax "=100.0, " mm Ymin "=0.0, "mm Ymax "=267.9, " mm Zmin"=0.0, "mm Zmax "=77.0, "Schritte oder mm Umin (0)"=0.0, "Schritte oder mm Umax (0)"=0.0, "Schritte oder mm Cmin (0)"=0.0, "Schritte oder mm Cmax (0)"=0.0, "Schritte oder mm Amin (0)"=0.0, "Schritte oder mm Amax (0)"=0.0, "Schritte oder mm Bmin (0)"=0.0, "Schritte oder mm Bmax (0)"=0.0} ("X,Y,Z Value Limits")) -> ()
              }
              frame "Manual Control" {
                n132 = flat-sequence {
                  tunnel: [w148] -> w138
                  tunnel: w137 -> [w148]
                  tunnel: [w147] -> w135
                  tunnel: w134 -> [w147]
                  tunnel: [w156] -> w145
                  tunnel: [w155] -> w144
                  tunnel: [w154] -> w143
                  tunnel: [w153] -> w142
                  tunnel: [w152] -> w139
                  tunnel: w138 -> [w152]
                  tunnel: [w151] -> w136
                  tunnel: w135 -> [w151]
                  tunnel: [w166] -> w141
                  tunnel: w145 -> [w165]
                  tunnel: w144 -> [w164]
                  tunnel: w143 -> [w163]
                  tunnel: w142 -> [w162]
                  tunnel: w139 -> [w161]
                  tunnel: w136 -> [w158]
                  tunnel: [w160] -> w130
                  tunnel: [w159] -> w126
                  tunnel: w141 -> [w169]
                  tunnel: [w168] -> w131
                  tunnel: w130 -> [w168]
                  tunnel: [w167] -> w127
                  tunnel: w126 -> [w167]
                  tunnel: cluster{u16, u16, dbl, bool} {36, 1, 0.0, TRUE} -> [w173]
                  tunnel: [w172] -> w132
                  tunnel: w131 -> [w172]
                  tunnel: [w171] -> w128
                  tunnel: w127 -> [w171]
                  tunnel: [w175] -> w133
                  tunnel: w132 -> [w175]
                  tunnel: [w174] -> w129
                  tunnel: w128 -> [w174]
                  frame #0 {
                    w149 = TRUE ("Moving")
                    n133 = Not(x=w149) -> (.not. x?=w150:bool)
                    n134 = local write "Moving"(w149) -> ()
                    n135 = local write "Stopped"(w150) -> ()
                  }
                  frame #1 {
                    n136 = local read "Movement"() -> (w157:T2)
                    n137 = Unbundle(w157) -> ("Axis"=w156:u8, "Direction(To/From)"=w155:u8, "Speed in mm/s\n (5)[0,025-20]"=w154:sgl, "IV6"=w153:bool)
                  }
                  frame #2 {
                    n138 = call <userlib>:"SubVI_Einzelschritte_IF5_IF6.vi"("VISA resource name in"=w158, "Achsen-Wahl (X)"=w165, "Geschwindigkeit\nin mm/s (5)[0,025-20]"=w163, "IF5=F/IF6=T\n(IF6=T) in"=w162, "error in"=w161, "Richtung (vEw)"=w164) -> ("VISA resource name out"=w160:refnum<visa-resource-name>, "Koordinaten IF6"=w166:T8, "error out"=w159:errorcluster)  [unwired: 3 in, 4 out]
                  }
                  frame #3 {
                    n139 = local write "Current Cordinates"(w169) -> ()
                    n140 = Wait (ms)(milliseconds to wait=u32 100) -> ()  [unwired: 1 out]
                  }
                  frame #4 {
                    n141 = local write "Movement"(w173) -> ()
                  }
                  frame #5 {
                    w178 = TRUE ("Moving")
                    n142 = Not(x=w178) -> (.not. x?=w177:bool)
                    n143 = local write "Stopped"(w178) -> ()
                    n144 = local write "Moving"(w177) -> ()
                    n145 = local write "Operation Done"("Manual movement of Platform" ("Status")) -> ()
                  }
                }
              }
              frame "Save Positions" {
                n146 = flat-sequence {
                  frame #0 {
                    n147 = local read "Current Cordinates"() -> (w185:T5)
                    n148 = local read "Position"() -> (w187:T4)
                    n149 = Unbundle(w185) -> ("X axis"=w182:sgl, "Y axis"=w183:sgl, "Z axis"=w184:sgl)  [unwired: 4 out]
                    n150 = Build Array(w182, w183, w184) -> (w186:sgl[])
                    n151 = case shown="\"Position 1\", Default" w187 {
                      tunnel: w186 -> [w188 w189 w190 w191 w192 w193 w194 w195 w196 w197]
                      frame "Position 1", Default {
                        n152 = local write "P1"(w188) -> ()
                      }
                      frame "Position 2" {
                        n153 = local write "P2"(w189) -> ()
                      }
                      frame "Position 3" {
                        n154 = local write "P3"(w190) -> ()
                      }
                      frame "Position 4" {
                        n155 = local write "P4"(w191) -> ()
                      }
                      frame "Position 5" {
                        n156 = local write "P5"(w192) -> ()
                      }
                      frame "Position 6" {
                        n157 = local write "P6"(w193) -> ()
                      }
                      frame "Position 7" {
                        n158 = local write "P7"(w194) -> ()
                      }
                      frame "Position 8" {
                        n159 = local write "P8"(w195) -> ()
                      }
                      frame "Position 9" {
                        n160 = local write "P9"(w196) -> ()
                      }
                      frame "Position 10" {
                        n161 = local write "P10"(w197) -> ()
                      }
                    }
                  }
                  frame #1 {
                    n162 = local write "Save"(FALSE ("Save Button")) -> ()
                    n163 = local write "Operation Done"("Position cordinates saved" ("Operation Done")) -> ()
                  }
                }
              }
              frame "Reset Position" {
                n164 = flat-sequence {
                  frame #0 {
                    n165 = local read "Position"() -> (w203:T4)
                    n166 = case shown="\"Position 10\"" w203 {
                      tunnel: dbl[] [0.0, 0.0, 0.0] ("P1") -> [w205 w206 w207 w208 w209 w210 w211 w212 w213 w214]
                      frame "Position 1", Default {
                        n167 = local write "P1"(w205) -> ()
                      }
                      frame "Position 2" {
                        n168 = local write "P2"(w206) -> ()
                      }
                      frame "Position 3" {
                        n169 = local write "P3"(w207) -> ()
                      }
                      frame "Position 4" {
                        n170 = local write "P4"(w208) -> ()
                      }
                      frame "Position 5" {
                        n171 = local write "P5"(w209) -> ()
                      }
                      frame "Position 6" {
                        n172 = local write "P6"(w210) -> ()
                      }
                      frame "Position 7" {
                        n173 = local write "P7"(w211) -> ()
                      }
                      frame "Position 8" {
                        n174 = local write "P8"(w212) -> ()
                      }
                      frame "Position 9" {
                        n175 = local write "P9"(w213) -> ()
                      }
                      frame "Position 10" {
                        n176 = local write "P10"(w214) -> ()
                      }
                    }
                  }
                  frame #1 {
                    n177 = local write "Reset"(FALSE ("Reset")) -> ()
                    n178 = local write "Operation Done"("The selected position is reset" ("Operation Done")) -> ()
                  }
                }
              }
              frame "Reset All" {
                n179 = flat-sequence {
                  frame #0 {
                    w220 = dbl[] [0.0, 0.0, 0.0] ("P1")
                    n180 = local write "P1"(w220) -> ()
                    n181 = local write "P2"(w220) -> ()
                    n182 = local write "P3"(w220) -> ()
                    n183 = local write "P4"(w220) -> ()
                    n184 = local write "P5"(w220) -> ()
                    n185 = local write "P6"(w220) -> ()
                    n186 = local write "P7"(w220) -> ()
                    n187 = local write "P8"(w220) -> ()
                    n188 = local write "P9"(w220) -> ()
                    n189 = local write "P10"(w220) -> ()
                    n190 = local write "Steps(mm)"(w220) -> ()
                  }
                  frame #1 {
                    n191 = local write "Reset All"(FALSE ("Reset all Positions")) -> ()
                    n192 = local write "Operation Done"("Reset all positions" ("Operation Done")) -> ()
                  }
                }
              }
              frame "Go Position" {
                n193 = flat-sequence {
                  tunnel: [w235] -> w226
                  tunnel: [w234] -> w225
                  tunnel: w230 -> [w237]
                  tunnel: w229 -> [w236]
                  tunnel: w226 -> [w261]
                  tunnel: w225 -> [w260]
                  tunnel: [w261] -> w224
                  tunnel: [w260] -> w223
                  tunnel: [w266] -> w227
                  tunnel: [w267] -> w228
                  tunnel: w224 -> [w267]
                  tunnel: w223 -> [w266]
                  frame #0 {
                    w233 = TRUE ("Moving")
                    n194 = local write "Moving"(w233) -> ()
                    n195 = local read "Position"() -> (w245:T4)
                    n196 = case shown="\"Position 10\"" w245 {
                      tunnel: [w246 w247 w248 w249 w250 w251 w252 w253 w254 w255] -> w243
                      frame "Position 1", Default {
                        n197 = local read "P1"() -> (w246:dbl[])
                      }
                      frame "Position 2" {
                        n198 = local read "P2"() -> (w247:dbl[])
                      }
                      frame "Position 3" {
                        n199 = local read "P3"() -> (w248:dbl[])
                      }
                      frame "Position 4" {
                        n200 = local read "P4"() -> (w249:dbl[])
                      }
                      frame "Position 5" {
                        n201 = local read "P5"() -> (w250:dbl[])
                      }
                      frame "Position 6" {
                        n202 = local read "P6"() -> (w251:dbl[])
                      }
                      frame "Position 7" {
                        n203 = local read "P7"() -> (w252:dbl[])
                      }
                      frame "Position 8" {
                        n204 = local read "P8"() -> (w253:dbl[])
                      }
                      frame "Position 9" {
                        n205 = local read "P9"() -> (w254:dbl[])
                      }
                      frame "Position 10" {
                        n206 = local read "P10"() -> (w255:dbl[])
                      }
                    }
                    n207 = Not(x=w233) -> (.not. x?=w232:bool)
                    n208 = local write "Stopped"(w232) -> ()
                    n209 = local read "Speed"() -> (w239:dbl)
                    n210 = local read "Current Cordinates"() -> (w242:T5)
                    n211 = Bundle(0, "Speed"=w239, 0) -> (w238:cluster{i32, "Speed":dbl, i32})  [unwired: 1 in]
                    n212 = call <userlib>:"SubVI_Punkt_anfahren_IF5_IF6.vi"("Angehängtes Array"=w243, "error in"=w236, "Koordinaten in IF6"=w242, "Geschwindigkeiten"=w238, "VISA resource name in"=w237) -> ("error out"=w234:errorcluster, "Koordinaten out IF6"=w244:T8, "VISA resource name in 2"=w235:refnum<visa-resource-name>)  [unwired: 1 in]
                    n213 = local write "Current Cordinates"(w244) -> ()
                  }
                  frame #1 {
                    w256 = TRUE ("Moving")
                    n214 = local write "Go To"(FALSE ("Go To")) -> ()
                    n215 = local write "Stopped"(w256) -> ()
                    n216 = Not(x=w256) -> (.not. x?=w257:bool)
                    n217 = local write "Moving"(w257) -> ()
                    n218 = local write "Operation Done"("Go to the selected position" ("Operation Done")) -> ()
                  }
                  frame #2 {
                    n219 = property on="Multiple Control" class="TabCtl (strict)"() -> ("Pages"=w262:refnum<vi>[])  [unwired: 2 in, 2 out]
                    n220 = Index Array(array=w262, index=1) -> (element=w263:refnum<vi>)
                    n221 = property class="Page"(reference=w263, "PageEnb"=T6."Page Enabled" ("Page Enabled State")) -> ()  [unwired: 1 in, 2 out]
                  }
                }
              }
              frame "Import Cordinates" {
                n222 = flat-sequence {
                  frame #0 {
                    n223 = local read "File Path"() -> (w281:path)
                    n224 = call "Dekoder Batch Speicher.vi"("Batchfeld Speicher"=w281) -> ("P9"=w271:dbl[], "P10"=w272:dbl[], "P1"=w273:dbl[], "P2"=w274:dbl[], "P8"=w275:dbl[], "P3"=w276:dbl[], "P4"=w277:dbl[], "P7"=w280:dbl[], "P6"=w278:dbl[], "P5"=w279:dbl[])  [unwired: 5 in]
                    n225 = local write "P9"(w271) -> ()
                    n226 = local write "P10"(w272) -> ()
                    n227 = local write "P1"(w273) -> ()
                    n228 = local write "P2"(w274) -> ()
                    n229 = local write "P8"(w275) -> ()
                    n230 = local write "P3"(w276) -> ()
                    n231 = local write "P4"(w277) -> ()
                    n232 = local write "P5"(w279) -> ()
                    n233 = local write "P6"(w278) -> ()
                    n234 = local write "P7"(w280) -> ()
                  }
                  frame #1 {
                    n235 = local write "Import"(FALSE ("Import")) -> ()
                    n236 = local write "Operation Done"("Import the position cordinates" ("Operation Done")) -> ()
                  }
                }
              }
              frame "Export Cordinates" {
                n237 = flat-sequence {
                  frame #0 {
                    n238 = Two Button Dialog(message="Copy the values to ? ", 1:"New File" ("F button name (\"Cancel\")"), 2:"Existing File" ("T button name (\"OK\")")) -> (T button?=w287:bool)
                    n239 = case shown="True" w287 {
                      frame False {
                        n240 = local read "P10"() -> (w297:dbl[])
                        n241 = local read "P1"() -> (w303:dbl[])
                        n242 = local read "P2"() -> (w302:dbl[])
                        n243 = local read "P3"() -> (w301:dbl[])
                        n244 = local read "P4"() -> (w300:dbl[])
                        n245 = local read "P5"() -> (w299:dbl[])
                        n246 = local read "P6"() -> (w298:dbl[])
                        n247 = local read "P7"() -> (w294:dbl[])
                        n248 = local read "P8"() -> (w295:dbl[])
                        n249 = local read "P9"() -> (w296:dbl[])
                        n250 = Build Array(w303, w302, w301, w300, w299, w298, w294, w295, w296, w297) -> (w291:dbl[][])
                        n251 = call-poly <vilib>:"Write To Spreadsheet File.vi"("format (%.3f)"="%.6f", "2D data"=w291) -> ("new file path (Not A Path if cancelled)"=w293:path)  [unwired: 6 in]
                        n252 = local write "File Path"(w293) -> ()
                      }
                      frame True {
                        n253 = local read "P10"() -> (w305:dbl[])
                        n254 = local read "P1"() -> (w306:dbl[])
                        n255 = local read "P2"() -> (w307:dbl[])
                        n256 = local read "P3"() -> (w308:dbl[])
                        n257 = local read "P4"() -> (w309:dbl[])
                        n258 = local read "P5"() -> (w310:dbl[])
                        n259 = local read "P6"() -> (w311:dbl[])
                        n260 = local read "P7"() -> (w312:dbl[])
                        n261 = local read "P8"() -> (w313:dbl[])
                        n262 = local read "P8"() -> (w314:dbl[])
                        n263 = Build Array(w306, w307, w308, w309, w310, w311, w312, w313, w314, w305) -> (w315:dbl[][])
                        n264 = local read "File Path"() -> (w304:path)
                        n265 = call-poly <vilib>:"Write To Spreadsheet File.vi"("format (%.3f)"="%.6f", "2D data"=w315, "file path (dialog if empty)"=w304) -> ()  [unwired: 5 in, 1 out]
                      }
                    }
                  }
                  frame #1 {
                    n266 = local write "Export"(FALSE ("Export")) -> ()
                    n267 = local write "Operation Done"("Export the position cordinates" ("Operation Done")) -> ()
                  }
                }
              }
              frame "Home Position" {
                n268 = flat-sequence {
                  tunnel: [w329] -> w326
                  tunnel: w325 -> [w329]
                  tunnel: [w328] -> w324
                  tunnel: w323 -> [w328]
                  tunnel: w326 -> [w336]
                  tunnel: w324 -> [w335]
                  tunnel: [w334] -> w321
                  tunnel: [w333] -> w319
                  tunnel: [w341] -> w322
                  tunnel: w321 -> [w341]
                  tunnel: [w340] -> w320
                  tunnel: w319 -> [w340]
                  frame #0 {
                    w330 = TRUE ("Moving")
                    n269 = Not(x=w330) -> (.not. x?=w331:bool)
                    n270 = local write "Moving"(w330) -> ()
                    n271 = local write "Stopped"(w331) -> ()
                  }
                  frame #1 {
                    w338 = u16 6 items=["X-Achse", "Y-Achse", "Z-Achse", "X- und Y-Achse", "X- und Z-Achse", "Y- und Z-Achse", "X, Y und Z-Achse", "U-Achse", "keine Achse"] ("Beteiligte Achsen (X,Y,Z,U)")
                    n272 = call "SubVI_Home_XYZU_IF5_IF6.vi"("VISA resource name in"=w335, "Beteiligte Achsen (X,Y,Z,U)"=w338, "Geschwindigkeiten"=T7 {"Geschwindigkeit X in mm/s\n(5) [0,025-15]"=10.0, "Geschwindigkeit Y in mm/s\n(5) [0,025-15]"=10.0, "Geschwindigkeit Z in mm/s\n(5) [0,025-15]"=10.0, "GeschwindigkeitU in mm/s\n(5) [0,025-15]"=2.0}, "IF5=F/IF6=T\n(IF6=T) in"=TRUE ("IF5=F/IF6=T\n(IF6=T) in"), "error in"=w336) -> ("VISA resource name out"=w334:refnum<visa-resource-name>, "Koordinaten IF6"=w337:T8, "error out"=w333:errorcluster)  [unwired: 3 in, 5 out]
                    n273 = local write "Current Cordinates"(w337) -> ()
                  }
                  frame #2 {
                    w344 = FALSE ("Moving")
                    n274 = Not(x=w344) -> (.not. x?=w345:bool)
                    n275 = local write "Moving"(w344) -> ()
                    n276 = local write "Stopped"(w345) -> ()
                    n277 = local write "Home Position"(FALSE ("Go To")) -> ()
                    n278 = local write "Operation Done"("The platform is taken to home position (0,0,0)" ("Operation Done")) -> ()
                  }
                }
              }
              frame "Load Sequence" {
                n279 = flat-sequence {
                  frame #0 {
                    n280 = local read "File  Select"() -> (w350:path)
                    n281 = call-poly <vilib>:"Read From Spreadsheet File.vi"("file path (dialog if empty)"=w350) -> ("all rows"=w349:string[][])  [unwired: 6 in, 4 out]
                    n282 = local write "Sequence"(w349) -> ()
                  }
                  frame #1 {
                    n283 = local write "Load Sequence"(FALSE ("Load Sequence")) -> ()
                    n284 = local write "Operation Done"("Sequence loaded" ("Status")) -> ()
                  }
                }
              }
              frame "Clear Sequence" {
                n285 = flat-sequence {
                  frame #0 {
                    n286 = Initialize Array("" ("element")) -> (w356:string[][])  [unwired: 2 in]
                    n287 = local write "Sequence"(w356) -> ()
                  }
                  frame #1 {
                    n288 = local write "Clear Sequence"(FALSE ("Clear Sequence")) -> ()
                    n289 = local write "Operation Done"("Sequence cleared" ("Status")) -> ()
                  }
                }
              }
              frame "Clear SensorReadings" {
                n290 = flat-sequence {
                  frame #0 {
                    n291 = local read "Clear Sensor Readings"() -> (w365:bool)
                    n292 = Initialize Array("" ("element")) -> (w366:string[][])  [unwired: 2 in]
                    n293 = local write "ED32i_output"(w366) -> ()
                    n294 = local write "ED33_output"(w366) -> ()
                    n295 = call "Sensor_Read.vi"("Clear"=w365) -> ()  [unwired: 8 in, 3 out]
                    n296 = property on="ED32i" class="WFChart (strict)"("History Data"=cluster{"Array 4[0]":i32, "Array 4[1]":i32}[] []) -> ()  [unwired: 2 in, 2 out]
                    n297 = property on="ED33" class="WFChart (strict)"("History Data"=i32[] []) -> ()  [unwired: 2 in, 2 out]
                  }
                  frame #1 {
                    n298 = local write "Clear Sensor Readings"(FALSE ("Clear Sensor Readings")) -> ()
                    n299 = local write "Operation Done"("Cleared sensor readings" ("Operation Done")) -> ()
                  }
                }
              }
              frame "Set Speed" {
                n300 = flat-sequence {
                  frame #0 {
                    n301 = local read "Current Sequence"() -> (w373:string[])
                    n302 = Index Array(array=w373, index=1) -> (element=w375:string)
                    n303 = Fract/Exp String To Number(string=w375) -> (number=w376:dbl)  [unwired: 3 in, 1 out]
                    n304 = local write "Speed"(w376) -> ()
                  }
                  frame #1 {
                    n305 = local write "Operation Done"("Speed Set") -> ()
                  }
                }
              }
              frame "Set Powersupply" {
                n306 = flat-sequence {
                  frame #0 {
                    n307 = local read "Current Sequence"() -> (w381:string[])
                    n308 = local read "Port for Powersupply"() -> (w387:refnum<visa-resource-name>)
                    n309 = Index Array(array=w381, index=1 ("Index")) -> (element=w383:string)
                    n310 = Concatenate Strings(w383, "\r") -> (w385:string)
                    n311 = call "Serial_com_powersupply für Funktion.vi"("VISA resource name"=w387, "write"=TRUE, "string to write"=w385) -> ()  [unwired: 6 in, 2 out]
                  }
                  frame #1 {
                    n312 = local read "Port for Write Head"() -> (w389:refnum<visa-resource-name>)
                    n313 = Concatenate Strings("GPV 6" ("string"), "\r") -> (w391:string)
                    n314 = call "Serial_com_powersupply für Funktion.vi"("VISA resource name"=w389, "write"=TRUE, "string to write"=w391) -> ()  [unwired: 6 in, 2 out]
                  }
                  frame #2 {
                    n315 = local write "Operation Done"("Powersupply Set") -> ()
                  }
                }
              }
              frame "Batch Position" {
                n316 = flat-sequence {
                  tunnel: [w402] -> w397
                  tunnel: [w401] -> w396
                  tunnel: w395 -> [w400]
                  tunnel: w394 -> [w399]
                  frame #0 {
                    n317 = local read "Current Sequence"() -> (w403:string[])
                    n318 = Index Array(array=w403, index=1) -> (element=w405:string)
                    n319 = case shown="\"Position 1\", Default" w405 {
                      tunnel: [w413 w414 w415 w416 w417 w418 w419 w420 w421 w422] -> w406
                      frame "Position 1", Default {
                        n320 = local read "P1"() -> (w413:dbl[])
                      }
                      frame "Position 2" {
                        n321 = local read "P2"() -> (w414:dbl[])
                      }
                      frame "Position 3" {
                        n322 = local read "P3"() -> (w415:dbl[])
                      }
                      frame "Position 4" {
                        n323 = local read "P4"() -> (w416:dbl[])
                      }
                      frame "Position 5" {
                        n324 = local read "P5"() -> (w417:dbl[])
                      }
                      frame "Position 6" {
                        n325 = local read "P6"() -> (w418:dbl[])
                      }
                      frame "Position 7" {
                        n326 = local read "P7"() -> (w419:dbl[])
                      }
                      frame "Position 8" {
                        n327 = local read "P8"() -> (w420:dbl[])
                      }
                      frame "Position 9" {
                        n328 = local read "P9"() -> (w421:dbl[])
                      }
                      frame "Position 10" {
                        n329 = local read "P10"() -> (w422:dbl[])
                      }
                    }
                    n330 = local read "Speed"() -> (w411:dbl)
                    n331 = Bundle(1, "Speed"=w411, 1) -> (w412:cluster{i32, "Speed":dbl, i32})  [unwired: 1 in]
                    n332 = local read "Current Cordinates"() -> (w407:T5)
                    n333 = call <userlib>:"SubVI_Punkt_anfahren_IF5_IF6.vi"("Angehängtes Array"=w406, "error in"=w400, "Koordinaten in IF6"=w407, "Geschwindigkeiten"=w412, "VISA resource name in"=w399) -> ("error out"=w401:errorcluster, "Koordinaten out IF6"=w408:T8, "VISA resource name in 2"=w402:refnum<visa-resource-name>)  [unwired: 1 in]
                    n334 = local write "Current Cordinates"(w408) -> ()
                  }
                  frame #1 {
                    n335 = local write "Operation Done"("Position Set") -> ()
                  }
                }
              }
              frame "Go Straight" {
                n336 = local read "ED32i Active?"() -> (w426:bool)
                n337 = local read "ED33 Active?"() -> (w425:bool)
                n338 = Or(x=w426, y=w425) -> (x .or. y?=w424:bool)
                n339 = case shown="True" w424 {
                  tunnel: w430 -> [w435 w468]
                  tunnel: w429 -> [w434 w471]
                  tunnel: [w433 w473] -> w428
                  tunnel: [w432 w470] -> w427
                  frame False {
                    n340 = flat-sequence {
                      tunnel: w435 -> [w449]
                      tunnel: [w451] -> w437
                      tunnel: [w450] -> w436
                      tunnel: w434 -> [w448]
                      tunnel: w437 -> [w465]
                      tunnel: [w465] -> w432
                      tunnel: [w464] -> w433
                      tunnel: w436 -> [w464]
                      frame #0 {
                        w455 = TRUE ("Moving")
                        n341 = local read "X axis"() -> (w444:enum16{"Left", "Right"})
                        n342 = local read "Y axis"() -> (w443:enum16{"Forward", "Backward"})
                        n343 = local read "Z axis"() -> (w442:enum16{"Up", "Down"})
                        n344 = case shown="\"Forward\", Default" w443 {
                          tunnel: [0 1] -> w446
                          frame "Forward", Default {
                          }
                          frame "Backward" {
                          }
                        }
                        n345 = case shown="\"Right\"" w444 {
                          tunnel: [1 0] -> w447
                          frame "Left", Default {
                          }
                          frame "Right" {
                          }
                        }
                        n346 = case shown="\"Down\"" w442 {
                          tunnel: [1 0] -> w445
                          frame "Up", Default {
                          }
                          frame "Down" {
                          }
                        }
                        n347 = local read "Steps(mm)"() -> (w441:dbl[])
                        n348 = local read "Current Sequence"() -> (w439:string[])
                        n349 = local read "Activate Sequence?"() -> (w453:bool)
                        n350 = Build Array (concatenate)(w441, w447, w446, w445) -> (w440:dbl[])
                        n351 = local read "Speed"() -> (w438:dbl)
                        n352 = Not(x=w455) -> (.not. x?=w454:bool)
                        n353 = local write "Moving"(w455) -> ()
                        n354 = local write "Stopped"(w454) -> ()
                        n355 = call "Go Straight.vi"("VISA resource name in"=w448, "Sequence Active"=w453, "array"=w439, "Speed"=w438, "Steps(mm)"=w440, "error in"=w449) -> ("VISA resource name out"=w451:refnum<visa-resource-name>, "Koordinaten IF6"=w452:T8, "error out"=w450:errorcluster)
                        n356 = local write "Current Cordinates"(w452) -> ()
                      }
                      frame #1 {
                        w466 = TRUE ("Stopped")
                        n357 = Not(x=w466) -> (.not. x?=w463:bool)
                        n358 = local write "Move Steps"(w463) -> ()
                        n359 = local write "Stopped"(w466) -> ()
                        n360 = local write "Moving"(w463) -> ()
                        n361 = local write "Operation Done"("Moved to corresponding position" ("Operation Done")) -> ()
                      }
                    }
                  }
                  frame True {
                    n362 = flat-sequence {
                      tunnel: w468 -> [w541]
                      tunnel: [w537] -> w472
                      tunnel: w471 -> [w536]
                      tunnel: [w535] -> w469
                      tunnel: [w553] -> w473
                      tunnel: w472 -> [w553]
                      tunnel: [w550] -> w470
                      tunnel: w469 -> [w550]
                      frame #0 {
                        w538 = TRUE ("Moving")
                        n363 = local read "Z axis"() -> (w532:enum16{"Up", "Down"})
                        n364 = local read "X axis"() -> (w534:enum16{"Left", "Right"})
                        n365 = local read "Y axis"() -> (w533:enum16{"Forward", "Backward"})
                        n366 = case shown="\"Backward\"" w533 {
                          tunnel: [0 1] -> w529
                          frame "Forward", Default {
                          }
                          frame "Backward" {
                          }
                        }
                        n367 = case shown="\"Right\"" w534 {
                          tunnel: [1 0] -> w530
                          frame "Left", Default {
                          }
                          frame "Right" {
                          }
                        }
                        n368 = case shown="\"Up\", Default" w532 {
                          tunnel: [1 0] -> w528
                          frame "Up", Default {
                          }
                          frame "Down" {
                          }
                        }
                        n369 = local read "Steps(mm)"() -> (w531:dbl[])
                        n370 = Build Array (concatenate)(w531, w530, w529, w528) -> (w527:dbl[])
                        n371 = local read "Activate Sequence?"() -> (w542:bool)
                        n372 = local read "Current Sequence"() -> (w543:string[])
                        n373 = call "Go Straight.vi"("VISA resource name in"=w536, "Sequence Active"=w542, "array"=w543, "Speed"=1, "Steps(mm)"=w527, "error in"=w541) -> ("VISA resource name out"=w535:refnum<visa-resource-name>, "Koordinaten IF6"=w540:T8, "error out"=w537:errorcluster)
                        n374 = Not(x=w538) -> (.not. x?=w539:bool)
                        n375 = local write "Moving"(w538) -> ()
                        n376 = local write "Current Cordinates"(w540) -> ()
                        n377 = local write "Stopped"(w539) -> ()
                      }
                      frame #1 {
                        w552 = TRUE ("Stopped")
                        n378 = Not(x=w552) -> (.not. x?=w551:bool)
                        n379 = local write "Stopped"(w552) -> ()
                        n380 = local write "Moving"(w551) -> ()
                        n381 = local write "Move Steps"(w551) -> ()
                      }
                    }
                    n382 = flat-sequence {
                      tunnel: w468 -> [w474]
                      frame #0 {
                        n383 = local read "ED32i Active?"() -> (w476:bool)
                        n384 = local read "ED33 Active?"() -> (w475:bool)
                        n385 = case shown="True" w476 {
                          selector: w476 -> [_ w478]
                          tunnel: w474 -> [_ w477]
                          frame False {
                          }
                          frame True {
                            n386 = while {
                              tunnel: w478 -> [w492]
                              tunnel: w477 -> [w491]
                              stop <- w490 stop-if-true
                              n387 = local read "Port for ED32i"() -> (w493:refnum<visa-resource-name>)
                              n388 = call "Sensor_Read.vi"("error in (no error)"=w491, "Port ED32i"=w493, "ED32i Active?"=w492, "ED33 Active?"=FALSE) -> ("ED32i_output"=w487:string[][])  [unwired: 5 in, 2 out]
                              n389 = local write "ED32i_output"(w487) -> ()
                              n390 = Index Array(array=w487, index (col)=0) -> (element=w486:string[])  [unwired: 1 in]
                              n391 = Index Array(array=w487, index (col)=1) -> (element=w484:string[])  [unwired: 1 in]
                              n392 = Index Array(array=w486) -> (element=w485:string)  [unwired: 1 in]
                              n393 = Index Array(array=w484) -> (element=w483:string)  [unwired: 1 in]
                              n394 = Decimal String To Number(string=w485) -> (number=w482:i32)  [unwired: 2 in, 1 out]
                              n395 = Decimal String To Number(string=w483) -> (number=w481:i32)  [unwired: 2 in, 1 out]
                              n396 = Bundle(w482, w481) -> (w480:cluster{i32, i32})  [unwired: 1 in]
                              n397 = local read "Stopped"() -> (w490:bool)
                              n398 = local write "ED32i"(w480) -> ()
                            }
                          }
                        }
                        n399 = case shown="True" w475 {
                          selector: w475 -> [_ w495]
                          tunnel: w474 -> [_ w494]
                          frame False {
                          }
                          frame True {
                            n400 = while {
                              tunnel: w495 -> [w503]
                              tunnel: w494 -> [w502]
                              stop <- w501 stop-if-true
                              n401 = local read "Port for ED33"() -> (w504:refnum<visa-resource-name>)
                              n402 = call "Sensor_Read.vi"("error in (no error)"=w502, "ED32i Active?"=FALSE, "ED33 Active?"=w503, "Port ED33"=w504) -> ("ED33_output"=w498:string[][])  [unwired: 5 in, 2 out]
                              n403 = local write "ED33_output"(w498) -> ()
                              n404 = Index Array(array=w498, index (col)=1) -> (element=w500:string[])  [unwired: 1 in]
                              n405 = Decimal String To Number(string=w500) -> (number=w497:i32[])  [unwired: 2 in, 1 out]
                              n406 = local read "Stopped"() -> (w501:bool)
                              n407 = local write "ED33"(w497) -> ()
                            }
                          }
                        }
                      }
                      frame #1 {
                        n408 = local read "ED32i Active?"() -> (w507:bool)
                        n409 = local read "ED33 Active?"() -> (w506:bool)
                        n410 = case shown="True" w507 {
                          selector: w507 -> [_ w511]
                          frame False {
                          }
                          frame True {
                            n411 = local read "Current Cordinates"() -> (w508:T5)
                            n412 = local read "ED32i_output"() -> (w510:string[][])
                            n413 = call "Sensor_Save.vi"("Current Cordinates"=w508, "ED32i Active?"=w511, "Cont/MM"="Continuous" ("Movement"), "ED33 Active?"=FALSE, "ED32i_output"=w510) -> ()  [unwired: 4 in]
                          }
                        }
                        n414 = case shown="True" w506 {
                          selector: w506 -> [_ w515]
                          frame False {
                          }
                          frame True {
                            n415 = local read "Current Cordinates"() -> (w513:T5)
                            n416 = local read "ED33_output"() -> (w516:string[][])
                            n417 = call "Sensor_Save.vi"("Current Cordinates"=w513, "ED32i Active?"=FALSE ("ED32i Active"), "Cont/MM"="Continuous" ("Movement"), "ED33 Active?"=w515, "ED33_output"=w516) -> ()  [unwired: 4 in]
                          }
                        }
                        n418 = local write "Operation Done"("Read values from sensors and values saved" ("Operation Done")) -> ()
                      }
                      frame #2 {
                        w525 = FALSE ("ED32i Active?")
                        n419 = property on="Multiple Control" class="TabCtl (strict)"() -> ("Pages"=w521:refnum<vi>[])  [unwired: 2 in, 2 out]
                        n420 = local write "ED32i Active?"(w525) -> ()
                        n421 = local write "ED33 Active?"(w525) -> ()
                        n422 = local write "Clear Sensor Readings"(TRUE ("Clear Sensor Readings")) -> ()
                        n423 = One Button Dialog(message="Sensor readings saved! ", button name ("OK")="OK") -> ()  [unwired: 1 out]
                        n424 = Index Array(array=w521, index=2) -> (element=w520:refnum<vi>)
                        n425 = property class="Page"(reference=w520, "PageEnb"=T6."Page Enabled" ("Page Enabled State")) -> ()  [unwired: 1 in, 2 out]
                      }
                    }
                    n426 = property on="Multiple Control" class="TabCtl (strict)"("Value"=enum32{"Position", "Sensors", "Results"}."Results" ("Tab Control")) -> ()  [unwired: 2 in, 2 out]
                  }
                }
              }
              frame "Set Steps" {
                n427 = flat-sequence {
                  frame #0 {
                    n428 = for {
                      N: 7 -> [_]
                      tunnel: [w577] -> w559 mode=indexing
                      i -> [w578]
                      n429 = local read "Current Sequence"() -> (w579:string[])
                      n430 = Increment(x=w578) -> (x+1=w581:i32)
                      n431 = Index Array(array=w579, index=w581) -> (element=w580:string)
                      n432 = Fract/Exp String To Number(string=w580) -> (number=w577:dbl)  [unwired: 3 in, 1 out]
                    }
                    n433 = Array To Cluster(array=w559) -> (cluster=w558:T9)
                    n434 = Unbundle(w558) -> ("[0]"=w560:dbl, "[1]"=w561:dbl, "[2]"=w562:dbl, "[3]"=w565:dbl, "[4]"=w566:dbl, "[5]"=w567:dbl)  [unwired: 3 out]
                    n435 = Bundle("[0]"=w560, "[1]"=w561, "[2]"=w562) -> (w563:cluster{"[0]":dbl, "[1]":dbl, "[2]":dbl})  [unwired: 1 in]
                    n436 = Cluster To Array(cluster=w563) -> (array=w564:dbl[])
                    n437 = case shown="1" w565 {
                      tunnel: [enum16{"Left", "Right"}."Right" enum16{"Left", "Right"}."Left"] -> w568
                      frame 0, Default {
                      }
                      frame 1 {
                      }
                    }
                    n438 = case shown="1" w566 {
                      tunnel: [enum16{"Forward", "Backward"}."Forward" enum16{"Forward", "Backward"}."Backward"] -> w570
                      frame 0, Default {
                      }
                      frame 1 {
                      }
                    }
                    n439 = case shown="1" w567 {
                      tunnel: [enum16{"Up", "Down"}."Down" enum16{"Up", "Down"}."Up"] -> w569
                      frame 0, Default {
                      }
                      frame 1 {
                      }
                    }
                    n440 = local write "Steps(mm)"(w564) -> ()
                    n441 = local write "X axis"(w568) -> ()
                    n442 = local write "Z axis"(w569) -> ()
                    n443 = local write "Y axis"(w570) -> ()
                  }
                  frame #1 {
                    n444 = local write "Operation Done"("Steps Set") -> ()
                  }
                }
              }
              frame "Set Count" {
                n445 = flat-sequence {
                  frame #0 {
                    n446 = local read "Current Sequence"() -> (w588:string[])
                    n447 = Index Array(array=w588, index=1) -> (element=w587:string)
                    n448 = Fract/Exp String To Number(string=w587) -> (number=w589:dbl)  [unwired: 3 in, 1 out]
                    n449 = local write "Count"(w589) -> ()
                  }
                  frame #1 {
                    n450 = local write "Operation Done"("Count Set") -> ()
                  }
                }
              }
              frame "Move & Measure" {
                n451 = local read "ED32i Active?"() -> (w596:bool)
                n452 = local read "ED33 Active?"() -> (w595:bool)
                n453 = Or(x=w596, y=w595) -> (x .or. y?=w591:bool)
                n454 = case shown="True" w591 {
                  tunnel: w593 -> [w598 w604]
                  tunnel: w594 -> [_ w603]
                  tunnel: [w598 w600] -> w592
                  frame False {
                  }
                  frame True {
                    n455 = local read "Count"() -> (w599:dbl)
                    n456 = for {
                      N: w599 -> [_]
                      tunnel: w604 -> [w644]
                      tunnel: w603 -> [w633]
                      tunnel: [w640] -> w601
                      w641 = TRUE
                      n457 = flat-sequence {
                        tunnel: w644 -> [w649]
                        tunnel: w633 -> [w648]
                        tunnel: [w647] -> w643
                        tunnel: [w646] -> w639
                        tunnel: w643 -> [w668]
                        tunnel: [w667] -> w640
                        tunnel: w639 -> [w667]
                        frame #0 {
                          n458 = local read "Steps(mm)"() -> (w645:dbl[])
                          n459 = local read "Y axis"() -> (w655:enum16{"Forward", "Backward"})
                          n460 = local read "Z axis"() -> (w656:enum16{"Up", "Down"})
                          n461 = local read "X axis"() -> (w657:enum16{"Left", "Right"})
                          n462 = case shown="\"Backward\"" w655 {
                            tunnel: [0 1] -> w659
                            frame "Forward", Default {
                            }
                            frame "Backward" {
                            }
                          }
                          n463 = case shown="\"Right\"" w657 {
                            tunnel: [1 0] -> w660
                            frame "Left", Default {
                            }
                            frame "Right" {
                            }
                          }
                          n464 = case shown="\"Up\", Default" w656 {
                            tunnel: [1 0] -> w658
                            frame "Up", Default {
                            }
                            frame "Down" {
                            }
                          }
                          n465 = Build Array (concatenate)(w645, w660, w659, w658) -> (w651:dbl[])
                          n466 = local read "Current Sequence"() -> (w652:string[])
                          n467 = local read "Activate Sequence?"() -> (w653:bool)
                          n468 = call "Go Straight.vi"("VISA resource name in"=w649, "Sequence Active"=w653, "array"=w652, "Speed"=1, "Steps(mm)"=w651, "error in"=w648) -> ("VISA resource name out"=w646:refnum<visa-resource-name>, "Koordinaten IF6"=w650:T8, "error out"=w647:errorcluster)
                          n469 = local write "Current Cordinates"(w650) -> ()
                        }
                        frame #1 {
                          n470 = local read "ED32i Active?"() -> (w670:bool)
                          n471 = local read "ED33 Active?"() -> (w669:bool)
                          n472 = case shown="True" w669 {
                            selector: w669 -> [_ w679]
                            tunnel: w668 -> [_ w677]
                            frame False {
                            }
                            frame True {
                              n473 = local read "Port for ED33"() -> (w678:refnum<visa-resource-name>)
                              n474 = call "Sensor_Read.vi"("error in (no error)"=w677, "ED32i Active?"=FALSE, "ED33 Active?"=w679, "Port ED33"=w678) -> ("ED33_output"=w674:string[][])  [unwired: 5 in, 2 out]
                              n475 = local write "ED33_output"(w674) -> ()
                              n476 = Index Array(array=w674, index (col)=1) -> (element=w676:string[])  [unwired: 1 in]
                              n477 = Decimal String To Number(string=w676, default (0L)=i64 0) -> (number=w673:i64[])  [unwired: 1 in, 1 out]
                              n478 = local write "ED33"(w673) -> ()
                            }
                          }
                          n479 = case shown="True" w670 {
                            selector: w670 -> [_ w693]
                            tunnel: w668 -> [_ w691]
                            frame False {
                            }
                            frame True {
                              n480 = local read "Port for ED32i"() -> (w692:refnum<visa-resource-name>)
                              n481 = call "Sensor_Read.vi"("error in (no error)"=w691, "Port ED32i"=w692, "ED32i Active?"=w693, "ED33 Active?"=FALSE) -> ("ED32i_output"=w682:string[][])  [unwired: 5 in, 2 out]
                              n482 = local write "ED32i_output"(w682) -> ()
                              n483 = Index Array(array=w682, index (col)=0) -> (element=w688:string[])  [unwired: 1 in]
                              n484 = Index Array(array=w682, index (col)=1) -> (element=w686:string[])  [unwired: 1 in]
                              n485 = Index Array(array=w688) -> (element=w687:string)  [unwired: 1 in]
                              n486 = Index Array(array=w686) -> (element=w685:string)  [unwired: 1 in]
                              n487 = Decimal String To Number(string=w687) -> (number=w684:i32)  [unwired: 2 in, 1 out]
                              n488 = Decimal String To Number(string=w685) -> (number=w683:i32)  [unwired: 2 in, 1 out]
                              n489 = Bundle(w684, w683) -> (w681:cluster{i32, i32})  [unwired: 1 in]
                              n490 = local write "ED32i"(w681) -> ()
                            }
                          }
                        }
                      }
                      n491 = local write "Current Status"("Move and measure") -> ()
                      n492 = Not(x=w641) -> (.not. x?=w642:bool)
                      n493 = local write "Moving"(w641) -> ()
                      n494 = local write "Stopped"(w642) -> ()
                      n495 = property on="Multiple Control" class="TabCtl (strict)"("Value"=enum32{"Position", "Sensors", "Results"}."Results" ("Tab Control")) -> ()  [unwired: 2 in, 2 out]
                      n496 = property on="Multiple Control" class="TabCtl (strict)"() -> ("Pages"=w637:refnum<vi>[])  [unwired: 2 in, 2 out]
                      n497 = Index Array(array=w637, index=2) -> (element=w636:refnum<vi>)
                      n498 = property class="Page"(reference=w636, "PageEnb"=T6."Page Enabled" ("Page Enabled State")) -> ()  [unwired: 1 in, 2 out]
                    }
                    n499 = flat-sequence {
                      tunnel: [w605] -> w602
                      tunnel: w601 -> [w605]
                      tunnel: w602 -> [w629]
                      tunnel: [w629] -> w600
                      frame #0 {
                        n500 = local read "ED32i Active?"() -> (w607:bool)
                        n501 = local read "ED33 Active?"() -> (w606:bool)
                        n502 = case shown="True" w606 {
                          selector: w606 -> [_ w615]
                          frame False {
                          }
                          frame True {
                            n503 = local read "Steps(mm)"() -> (w609:dbl[])
                            n504 = local read "Current Cordinates"() -> (w611:T5)
                            n505 = local read "ED33_output"() -> (w613:string[][])
                            n506 = Index Array(array=w609, index=1) -> (element=w608:dbl)
                            n507 = call "Sensor_Save.vi"("Min_move"=w608, "Current Cordinates"=w611, "ED32i Active?"=FALSE, "Cont/MM"="Move&Measure" ("Movement"), "ED33 Active?"=w615, "ED33_output"=w613) -> ()  [unwired: 3 in]
                          }
                        }
                        n508 = case shown="True" w607 {
                          selector: w607 -> [_ w623]
                          frame False {
                          }
                          frame True {
                            n509 = local read "Steps(mm)"() -> (w618:dbl[])
                            n510 = local read "Current Cordinates"() -> (w619:T5)
                            n511 = local read "ED32i_output"() -> (w621:string[][])
                            n512 = Index Array(array=w618, index=1) -> (element=w616:dbl)
                            n513 = call "Sensor_Save.vi"("Min_move"=w616, "Current Cordinates"=w619, "ED32i Active?"=w623, "Cont/MM"="Move&Measure" ("Movement"), "ED33 Active?"=FALSE, "ED32i_output"=w621) -> ()  [unwired: 3 in]
                          }
                        }
                      }
                      frame #1 {
                        w631 = TRUE
                        w628 = FALSE
                        n514 = Not(x=w631) -> (.not. x?=w630:bool)
                        n515 = local write "Stopped"(w631) -> ()
                        n516 = local write "ED33 Active?"(w628) -> ()
                        n517 = local write "ED32i Active?"(w628) -> ()
                        n518 = local write "Move & Measure"(w628) -> ()
                        n519 = local write "Clear Sensor Readings"(TRUE ("Clear Sensor Readings")) -> ()
                        n520 = local write "Moving"(w630) -> ()
                        n521 = local write "Operation Done"("Moved and Measured") -> ()
                        n522 = One Button Dialog(message="Sensor readings saved! ", button name ("OK")="OK") -> ()  [unwired: 1 out]
                      }
                    }
                  }
                }
              }
              frame "Read Sensors" {
                n523 = flat-sequence {
                  frame #0 {
                    n524 = local read "Current Sequence"() -> (w699:string[])
                    n525 = Index Array(array=w699, index=1) -> (element=w697:string)
                    n526 = case shown="\"ED33\"" w697 {
                      frame "ED32i", Default {
                        n527 = local write "ED32i Active?"(TRUE ("ED32i Active?")) -> ()
                      }
                      frame "ED33" {
                        n528 = local write "ED33 Active?"(TRUE ("ED33 Active?")) -> ()
                      }
                    }
                  }
                  frame #1 {
                    n529 = local write "Operation Done"("Sensor selected") -> ()
                  }
                }
              }
              frame "Write Pole" {
                n530 = local read "Port for Powersupply"() -> (w706:refnum<visa-resource-name>)
                n531 = local read "Current Sequence"() -> (w708:string[])
                n532 = local read "Port for Write Head"() -> (w707:refnum<visa-resource-name>)
                n533 = call "Write Pole.vi"("Fehler (Eingang)"=w705, "array"=w708, "Port for write head"=w707, "Port for Powersupply"=w706) -> ("Fehler (Ausgang)"=w704:errorcluster)
              }
            }
          }
          frame Error {
            n534 = Unbundle(w711) -> ("source"=w710:string)  [unwired: 2 out]
            n535 = One Button Dialog(message=w710) -> (true=w714:bool)  [unwired: 1 in]
            n536 = local write "Stop Program"(w714) -> ()
            n537 = local write "Stopped"(w714) -> ()
            n538 = local write "Current Status"("Force stop due to error" ("Status")) -> ()
          }
        }
        n539 = local read "Stop Program"() -> (w51:bool)
        n540 = flat-sequence {
          tunnel: [w73] -> w52
          tunnel: w53 -> [w72]
          frame #0 {
            n541 = local read "Current Status"() -> (w74:string)
            n542 = case shown="\"Waiting for next instruction\"" w74 {
              selector: w74 -> [w76 _]
              tunnel: [w76 w77] -> w73
              tunnel: w72 -> [_ w77]
              frame "Pause", Default {
                n543 = local write "Current Status"("Waiting for next instruction" ("Status")) -> ()
              }
              frame "Waiting for next instruction" {
              }
            }
          }
        }
        n544 = case shown="True" w51 {
          frame False {
          }
          frame True {
            w69 = FALSE ("Moving")
            n545 = local write "Moving"(w69) -> ()
            n546 = Not(x=w69) -> (.not. x?=w70:bool)
            n547 = local write "Stopped"(w70) -> ()
            n548 = local write "Operation Done"("Program Stopped!!!" ("Status")) -> ()
          }
        }
      }
    }
  }
  n549 = local write "Error Out"(w1) -> ()
  n550 = call <vilib>:"General Error Handler.vi"("error in (no error)"=w1) -> ()  [unwired: 10 in, 5 out]
